vi "Coral Controller.vi"(3 "error in":errorcluster) -> ()   [LabVIEW 2023]
doc: "This VI executes continuously carrying out the current operation and responding to updates or new operations. It will often contain the timing or control code that is difficult to place directly in TeleOp. This VI generally opens all sensors and motors and isolates the rest of the robot code from knowing how the operations are carried out."
uses:
  <vilib>/Rock Robotics/WPI/Framework/Completion Status.ctl
  Coral Setpoints.ctl
  Coral Operations.ctl
  Support Code/Teleop Util/Coral States.ctl
  Support Code/Teleop Util/Scoring Levels.ctl
  <vilib>/Rock Robotics/WPI/ThirdParty/REV Robotics/REVLib/Typedef/Spark MAX Idle Mode.ctl
  <vilib>/Rock Robotics/WPI/ThirdParty/REV Robotics/REVLib/Typedef/SPARK Closed Loop Slot.ctl
  <vilib>/Rock Robotics/SystemInterfaces/DIO/FPGA_DIOChannel.ctl
  <vilib>/Rock Robotics/WPI/ThirdParty/REV Robotics/REVLib/Typedef/Spark MAX Control Type.ctl
  da023379-89e9-4f2e-8a2f-b1c80103741f.vi
  <vilib>/Rock Robotics/WPI/ThirdParty/REV Robotics/REVLib/SubVI/Public/SPARK Open Brushless.vi
  <vilib>/Rock Robotics/WPI/ThirdParty/REV Robotics/REVLib/SubVI/Public/SPARK Configure Basic Idle Mode.vi
  <vilib>/Rock Robotics/WPI/ThirdParty/REV Robotics/REVLib/SubVI/Public/SPARK Configure Basic Inverted.vi
  <vilib>/Rock Robotics/WPI/ThirdParty/REV Robotics/REVLib/SubVI/Public/SPARK Configure Encoder Conversion Factors.vi
  <vilib>/Rock Robotics/WPI/ThirdParty/REV Robotics/REVLib/SubVI/Public/SPARK Configure Limit Switch Reverse.vi
  <vilib>/Rock Robotics/WPI/ThirdParty/REV Robotics/REVLib/SubVI/Public/SPARK Configure Soft Limit Forward.vi
  <vilib>/Rock Robotics/WPI/ThirdParty/REV Robotics/REVLib/SubVI/Public/SPARK Configure Soft Limit Reverse.vi
  <vilib>/Rock Robotics/WPI/ThirdParty/REV Robotics/REVLib/SubVI/Public/SPARK Configure Power Smart Current Limit.vi
  <vilib>/Rock Robotics/WPI/ThirdParty/REV Robotics/REVLib/SubVI/Public/SPARK Configure Closed Loop Miscellaneous.vi
  <vilib>/Rock Robotics/Network Tables/NT Write String.vi
  Framework/Robot Global Data.vi
  <vilib>/Rock Robotics/Network Tables/NT Read Number.vi
  <vilib>/Rock Robotics/WPI/ThirdParty/REV Robotics/REVLib/SubVI/Public/SPARK Get Encoder Status Position.vi
  <vilib>/Rock Robotics/WPI/ThirdParty/REV Robotics/REVLib/SubVI/Public/SPARK Get Device Status Output Current.vi
  <vilib>/Rock Robotics/WPI/ThirdParty/REV Robotics/REVLib/SubVI/Public/SPARK Get Encoder Status Velocity.vi
  <vilib>/Rock Robotics/Network Tables/NT Write Number.vi
  <vilib>/Rock Robotics/WPI/ThirdParty/REV Robotics/REVLib/Typedef/Spark MAX Limit Switch Polarity.ctl
  <vilib>/Rock Robotics/WPI/ThirdParty/REV Robotics/REVLib/SubVI/Public/SPARK Configure Limit Switch Forward.vi
  <vilib>/Rock Robotics/Network Tables/NT Write Boolean.vi
  <vilib>/Rock Robotics/WPI/ThirdParty/REV Robotics/REVLib/SubVI/Public/SPARK Configure Follower Mode From Ref.vi
panel:
  out "Detect DIO0?":bool=TRUE
  in  "sensor speed launcher 2":dbl=850.0
  out "Coral Seen":dbl(graph)
  out "Detect DIO2?":bool=TRUE
  out "Detect DIO1?":bool=TRUE
  in  "Arbitrary Feed Forward (0)":dbl=0.7
  out "End Time":dbl=0.4
  out "Current":dbl(graph)=11.245421245421245
  in  "Trapezoid Fly off?":bool
  out "Grounded Trapezoid":cluster{"Sensor Velocity":dbl, "Numeric":dbl}[](graph)=[{"Sensor Velocity"=-0.075857974588871, "Numeric"=0.0}, {"Sensor Velocity"=-0.0156947523355484, "Numeric"=300.0}, {"Sensor Velocity"=-1.0724748373031616, "Numeric"=600.0}, {"Sensor Velocity"=6.980241298675537, "Numeric"=900.0}, {"Sensor Velocity"=67.09114837646484, "Numeric"=1200.0}, {"Sensor Velocity"=197.5812530517578, "Numeric"=1500.0}, {"Sensor Velocity"=419.5848388671875, "Numeric"=1800.0}, {"Sensor Velocity"=710.8807983398438, "Numeric"=2100.0}, {"Sensor Velocity"=1095.191650390625, "Numeric"=2400.0}, {"Sensor Velocity"=1497.837890625, "Numeric"=2700.0}, {"Sensor Velocity"=1889.49267578125, "Numeric"=3000.0}, {"Sensor Velocity"=2250.2314453125, "Numeric"=2947.8500604629517}, {"Sensor Velocity"=2563.325927734375, "Numeric"=2647.8500604629517}, {"Sensor Velocity"=2824.191162109375, "Numeric"=2347.8500604629517}, {"Sensor Velocity"=3000.52685546875, "Numeric"=2047.8500604629512}, {"Sensor Velocity"=2896.772705078125, "Numeric"=1747.850060462952}, {"Sensor Velocity"=2896.772705078125, "Numeric"=1447.8500604629517}, {"Sensor Velocity"=2564.4833984375, "Numeric"=1147.8500604629512}, {"Sensor Velocity"=2022.881103515625, "Numeric"=847.8500604629517}, {"Sensor Velocity"=1387.4384765625, "Numeric"=547.8500604629517}, {"Sensor Velocity"=826.7198486328125, "Numeric"=247.8500604629512}, {"Sensor Velocity"=386.8534240722656, "Numeric"=0.0}, {"Sensor Velocity"=110.9880599975586, "Numeric"=0.0}]
  out "Sensor Experiment":bool
  out "Post-Trapezoid Sensor Position":dbl=-9.590681076049805
  out "Scoring Sequence Trapezoid":cluster{"Sensor Velocity":dbl, "Numeric":dbl}[](graph)=[{"Sensor Velocity"=0.0, "Numeric"=-0.0}, {"Sensor Velocity"=-7.134573459625244, "Numeric"=-300.0}, {"Sensor Velocity"=-7.134573459625244, "Numeric"=-600.0}, {"Sensor Velocity"=-41.63425827026367, "Numeric"=-900.0}, {"Sensor Velocity"=-125.5266342163086, "Numeric"=-1200.0}, {"Sensor Velocity"=-259.8109436035156, "Numeric"=-1500.0}, {"Sensor Velocity"=-446.01348876953125, "Numeric"=-1800.0}, {"Sensor Velocity"=-687.0809936523438, "Numeric"=-2100.0}, {"Sensor Velocity"=-1302.1033935546875, "Numeric"=-2400.0}, {"Sensor Velocity"=-1302.1033935546875, "Numeric"=-2700.0}, {"Sensor Velocity"=-1660.494384765625, "Numeric"=-3000.0}, {"Sensor Velocity"=-1997.8662109375, "Numeric"=-2704.006862640381}, {"Sensor Velocity"=-2354.501953125, "Numeric"=-2404.006862640381}, {"Sensor Velocity"=-2687.039794921875, "Numeric"=-2104.006862640381}, {"Sensor Velocity"=-2901.859130859375, "Numeric"=-1804.0068626403804}, {"Sensor Velocity"=-2966.857666015625, "Numeric"=-1504.006862640381}, {"Sensor Velocity"=-2838.606689453125, "Numeric"=-1204.0068626403809}, {"Sensor Velocity"=-1969.9622802734375, "Numeric"=-904.0068626403804}, {"Sensor Velocity"=-1969.9622802734375, "Numeric"=-604.0068626403809}, {"Sensor Velocity"=-1384.843505859375, "Numeric"=-304.00686264038086}, {"Sensor Velocity"=-874.3311767578125, "Numeric"=0.0}, {"Sensor Velocity"=-466.64947509765625, "Numeric"=0.0}]
  in  "Acceleration Max":dbl=15000.0
  in  "Velocity Max":dbl=5000.0
  out "Coral Seen":dbl
  out "Velocity Chart for Tuning":dbl(graph)=920.4789428710938
  in  "Launcher PID":T1={"P Gain"=0.0, "I Gain"=1e-06, "D Gain"=0.0, "F Gain"=0.0001, "I Zone"=0.0, "Min Output"=-0.5, "Max Output"=0.5}
  in  "Max I Accum":dbl=100.0
  in  "L4 PID Constant":T1={"P Gain"=0.0, "I Gain"=0.0, "D Gain"=0.0, "F Gain"=0.0, "I Zone"=0.0, "Min Output"=-0.8, "Max Output"=0.8}
  in  "coral threshold":dbl=10.0
  in  "Distance Decrease Grounded":dbl
  out "Command Timing":u32(graph)=7
  in  "Distance Decrease":dbl
  out "Intake Trapezoid Chart":cluster{"Sensor Velocity":dbl, "Numeric":dbl}[](graph)
  out "Position Chart (All Time)":cluster{"Sensor Position":dbl}(graph)={"Sensor Position"=-0.0436662957072258}
  out "Post Position Correction":dbl=-9.5556640625
  out "detect?":bool
  in  "sensor speed launcher":dbl=1250.0
  in  "launcher speed":dbl=1250.0
  in  "FF multiplier":dbl=0.39
  out "Pivot Chart":T2(graph)={"Sensor Velocity"=-4.928565979003906, "Arbitrary Feedforward"=-6.429}
  in  "Velocity PID Test":T1={"P Gain"=0.0002, "I Gain"=0.0, "D Gain"=0.0, "F Gain"=0.000165, "I Zone"=0.0, "Min Output"=-1.0, "Max Output"=1.0}
  in  "Positional PID Test":T1={"P Gain"=0.07, "I Gain"=0.0, "D Gain"=0.0, "F Gain"=0.0, "I Zone"=0.0, "Min Output"=-0.6, "Max Output"=0.6}
  in  "Intake Pivot Test":T1={"P Gain"=0.09, "I Gain"=0.0, "D Gain"=0.0, "F Gain"=-0.0, "I Zone"=0.0, "Min Output"=-0.8, "Max Output"=0.8}
  in  "detected speed (0)":dbl
  in  "FeedForward Constants":cluster{"kA":dbl, "kS":dbl, "kG":dbl, "kV":dbl}={"kA"=0.0, "kS"=0.0, "kG"=-0.57, "kV"=0.0}
  in  "intake setpoint":dbl=-0.95
  in  "Interactive Values":T3
  out "Current\nCmd":string="Started at  07:33:49.500\n: Immediate,  CS Grounded, SS Default"
  in  "Buttons":cluster{"Execute Cmd":bool, "Abort Cmd":bool}
  out "Command Timing":cluster{"Start Time (ms)":u32, "Iterations":i32}={"Start Time (ms)"=1054953, "Iterations"=0}
  out "Status":T7=enum."Aborted"
  # "old value 1250"
  # "irrelevant for now"
  # "sarah wuz here\nreasonable terms\nriyasonable terms"
  # "luke was here(maybe idk anymore)"
  # "intake speed: must be negative"
  # "launchee speed when intaking"
  # "Interactive Command: You may fill in the settings for a command\nand schedule it with the Execute button. You can observe and abort\nany command while fine tuning the code for the controller."
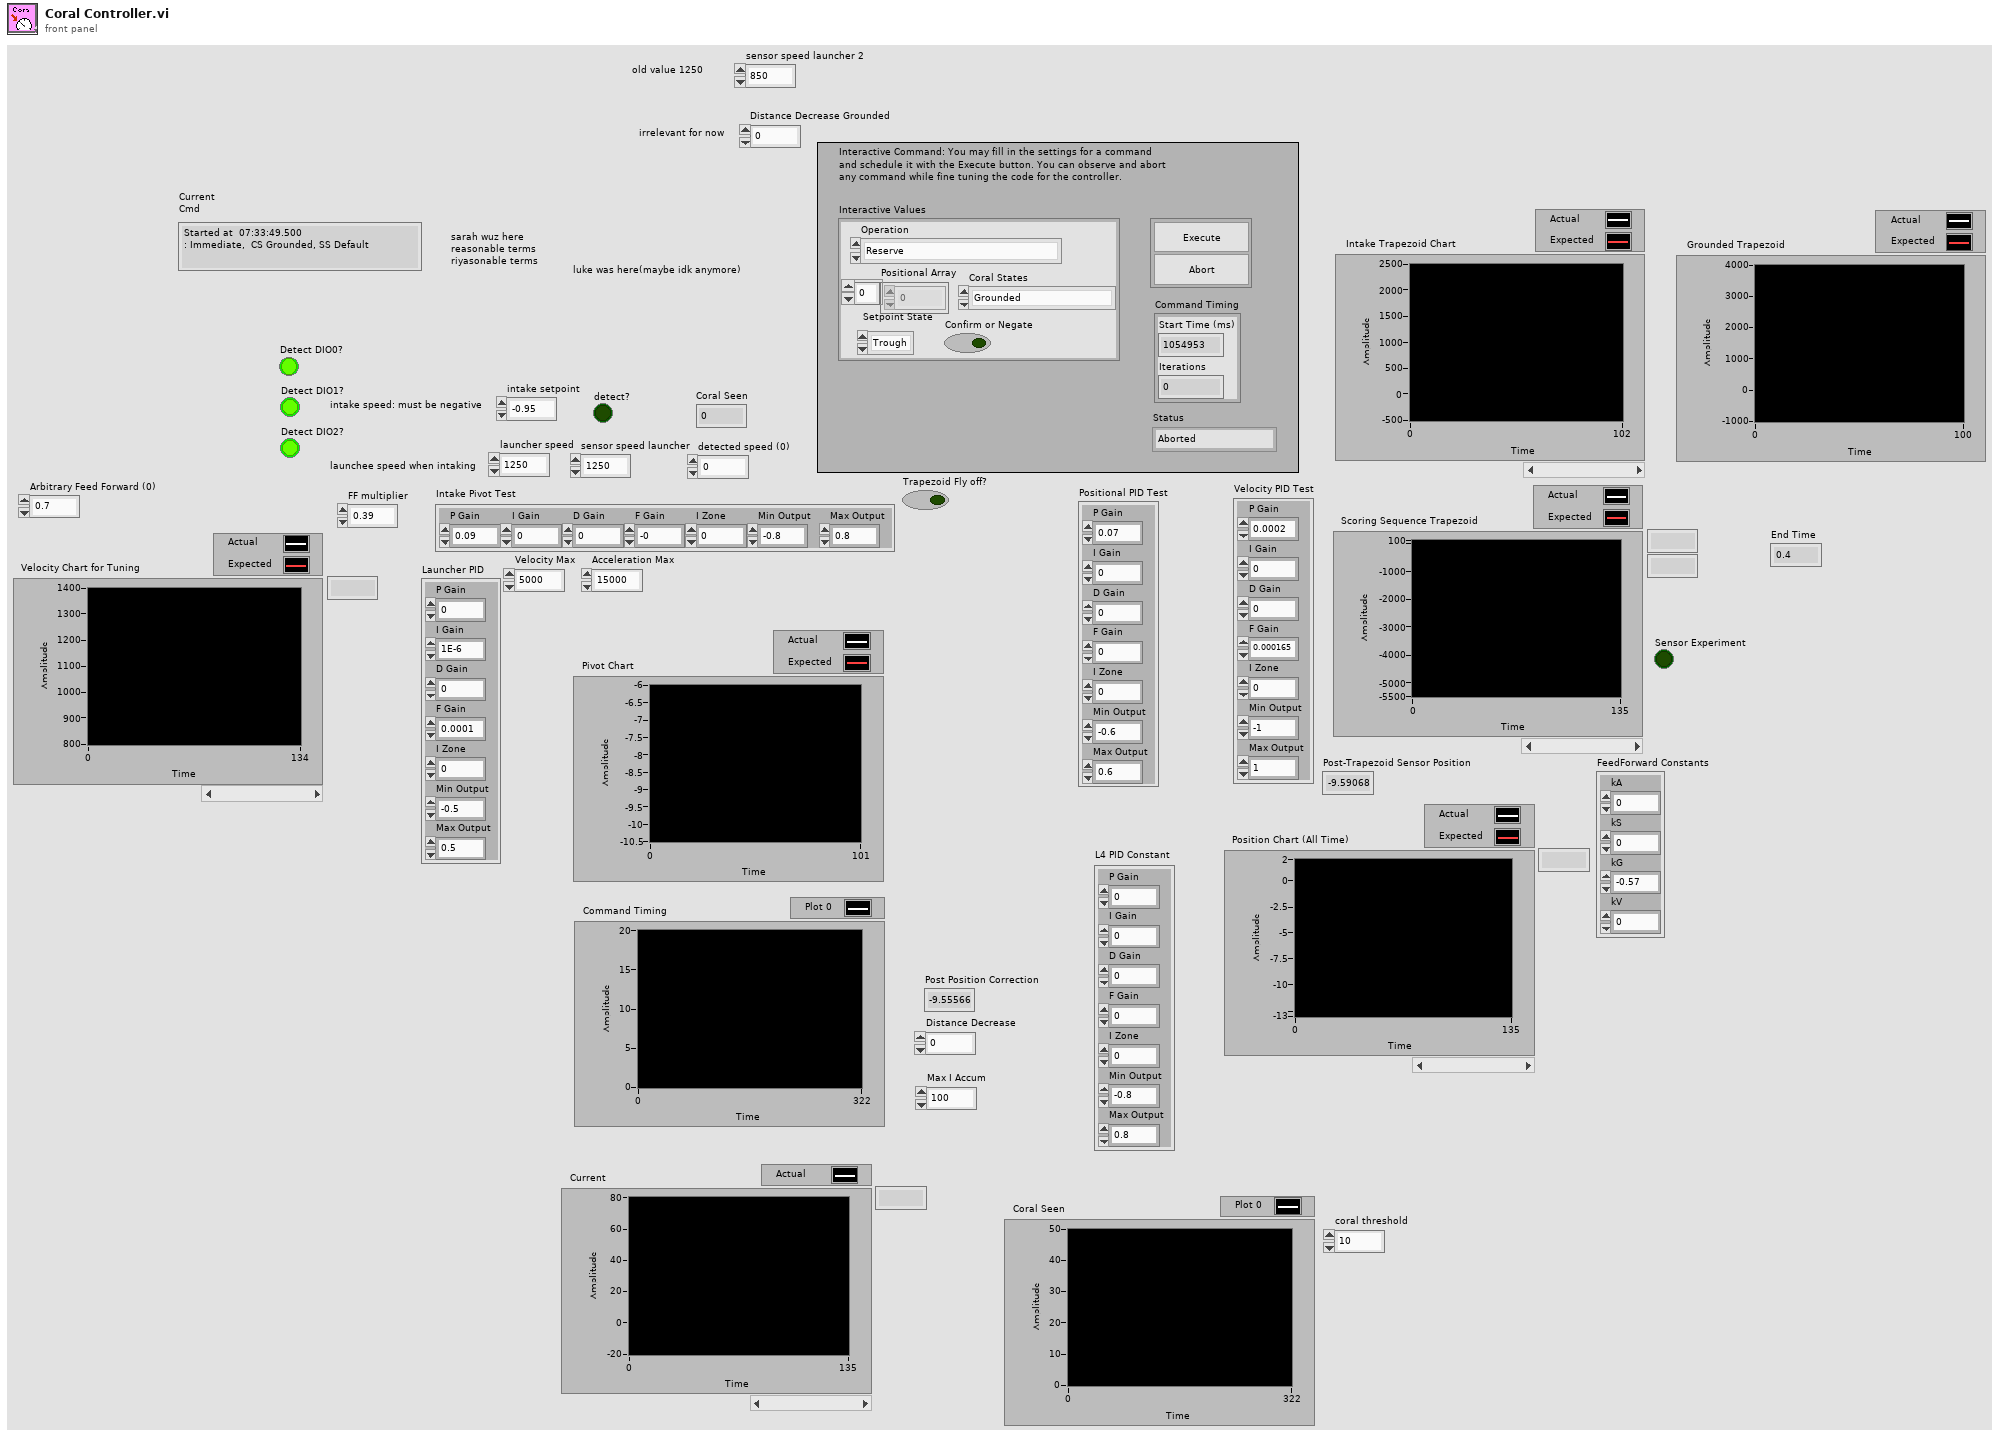
[diagram p1: front panel]
types:
  T1 = cluster{"P Gain":dbl, "I Gain":dbl, "D Gain":dbl, "F Gain":dbl, "I Zone":dbl, "Min Output":dbl, "Max Output":dbl}
  T2 = cluster{"Sensor Velocity":dbl, "Arbitrary Feedforward":dbl}
  T3 = typedef "Coral Setpoints.ctl" = cluster{"Operation":T4, "Coral States":T5, "Confirm or Negate":bool, "Positional Array":dbl[], "Setpoint State":T6}
  T4 = typedef "Coral Operations.ctl" = enum16{"Reserve", "Read Current", "Immediate", "Calibrate"}
  T5 = typedef "Coral States.ctl" = enum16{"Grounded", "Coral Intake", "Scoring Sequence", "Hold Position", "Score", "Manual Override", "Climb Safety Mode"}
  T6 = typedef "Scoring Levels.ctl" = enum16{"Trough", "L2", "L3", "L4", "Default"}
  T7 = typedef "Completion Status.ctl" = enum16{"Successful", "Aborted", "Incomplete"}
  T8 = typedef "FPGA_DIOChannel.ctl" = enum8{"DIO 0", "DIO 1", "DIO 2", "DIO 3", "DIO 4", "DIO 5", "DIO 6", "DIO 7", "DIO 8", "DIO 9", "DIO MXP 0", "DIO MXP 1", "DIO MXP 2", "DIO MXP 3", "DIO MXP 4", "DIO MXP 5", "DIO MXP 6", "DIO MXP 7", "DIO MXP 8", "DIO MXP 9", "DIO MXP 10", "DIO MXP 11", "DIO MXP 12", "DIO MXP 13", "DIO MXP 14", "DIO MXP 15", "SPI Port CS1", "SPI Port CS2", "SPI Port CS3", "SPI Port MISO", "SPI Port MOSI", "Invalid"}
  T9 = typedef "Spark MAX Idle Mode.ctl" = enum16{"Coast", "Brake"}
  T10 = typedef "SPARK Closed Loop Slot.ctl" = u16
  T11 = typedef "WPI_MotorControlDeviceRef.ctl" = cluster{"DeviceStatus":errorcluster, "Type":T12, "PWM":cluster{"PWM Channel":T13, "DeadBand":T14}, "CAN":cluster{"Device Number":u8, "SetOutput VI Ref":variant, "GetOutput VI Ref":variant, "Enable VI Ref":variant, "Disable VI Ref":variant, "Data":variant}, "Invert":bool, "DIO PWM":cluster{"PWM \"Enable\" Channel":T13, "DIOChannel":T8, "PWM Rate":dbl}}
  T12 = typedef "WPI_MotorControlType.ctl" = enum16{"PWM", "CAN", "DIO PWM"}
  T13 = typedef "FPGA_DIOPWMChannel.ctl" = enum8{"PWM 0", "PWM 1", "PWM 2", "PWM 3", "PWM 4", "PWM 5", "PWM 6", "PWM 7", "PWM 8", "PWM 9", "PWM MXP 0", "PWM MXP 1", "PWM MXP 2", "PWM MXP 3", "PWM MXP 4", "PWM MXP 5", "PWM MXP 6", "PWM MXP 7", "PWM MXP 8", "PWM MXP 9", "Invalid"}
  T14 = typedef "WPI_PWMDeadband.ctl" = cluster{"Name":string, "maxPositivePwm":i32, "minPositivePwm":i32, "centerPwm":i32, "maxNegativePwm":i32, "minNegativePwm":i32, "angularRange":u16}
  T15 = typedef "Command Status Info.ctl" = cluster{"Name":string, "Status":T7, "notifier out":T16}
  T16 = typedef "Completion Notifier.ctl" = refnum<notifier>
  T17 = typedef "WPI_DigitalInputDevRef.ctl" = cluster{"DevStatus":errorcluster, "DIO Channel":T8}
  T18 = cluster{"Current Command":T3, "Command Timing":cluster{"Start Time (ms)":u32, "Iterations":i32}, "Command Arguments":cluster{"Command Info":T15, "Description":string, "Default Command":T3, "queue out":refnum<queue>, "Subsystem Name":string}}
  T19 = typedef "Spark MAX Control Type.ctl" = enum16{"Percent VBus", "Voltage", "Velocity", "Position", "Smart Motion", "Current", "Smart Velocity", "MAXMotion Position", "MAXMotion Velocity"}
  T20 = typedef "Spark MAX Limit Switch Polarity.ctl" = enum16{"Normally Open", "Normally Closed"}
  T21 = cluster{"Setpoint Configs":cluster{"Scoring Setpoint":T6, "Position Setpoint":dbl, "Trapezoid":dbl[], "Score Power":dbl}[]}
  T22 = cluster{"Scoring Setpoint":T6, "Position Setpoint":dbl, "Trapezoid":dbl[], "Score Power":dbl}[]
  T23 = cluster{"Scoring Setpoint":T6, "Position Setpoint":dbl, "Trapezoid":dbl[], "Score Power":dbl}
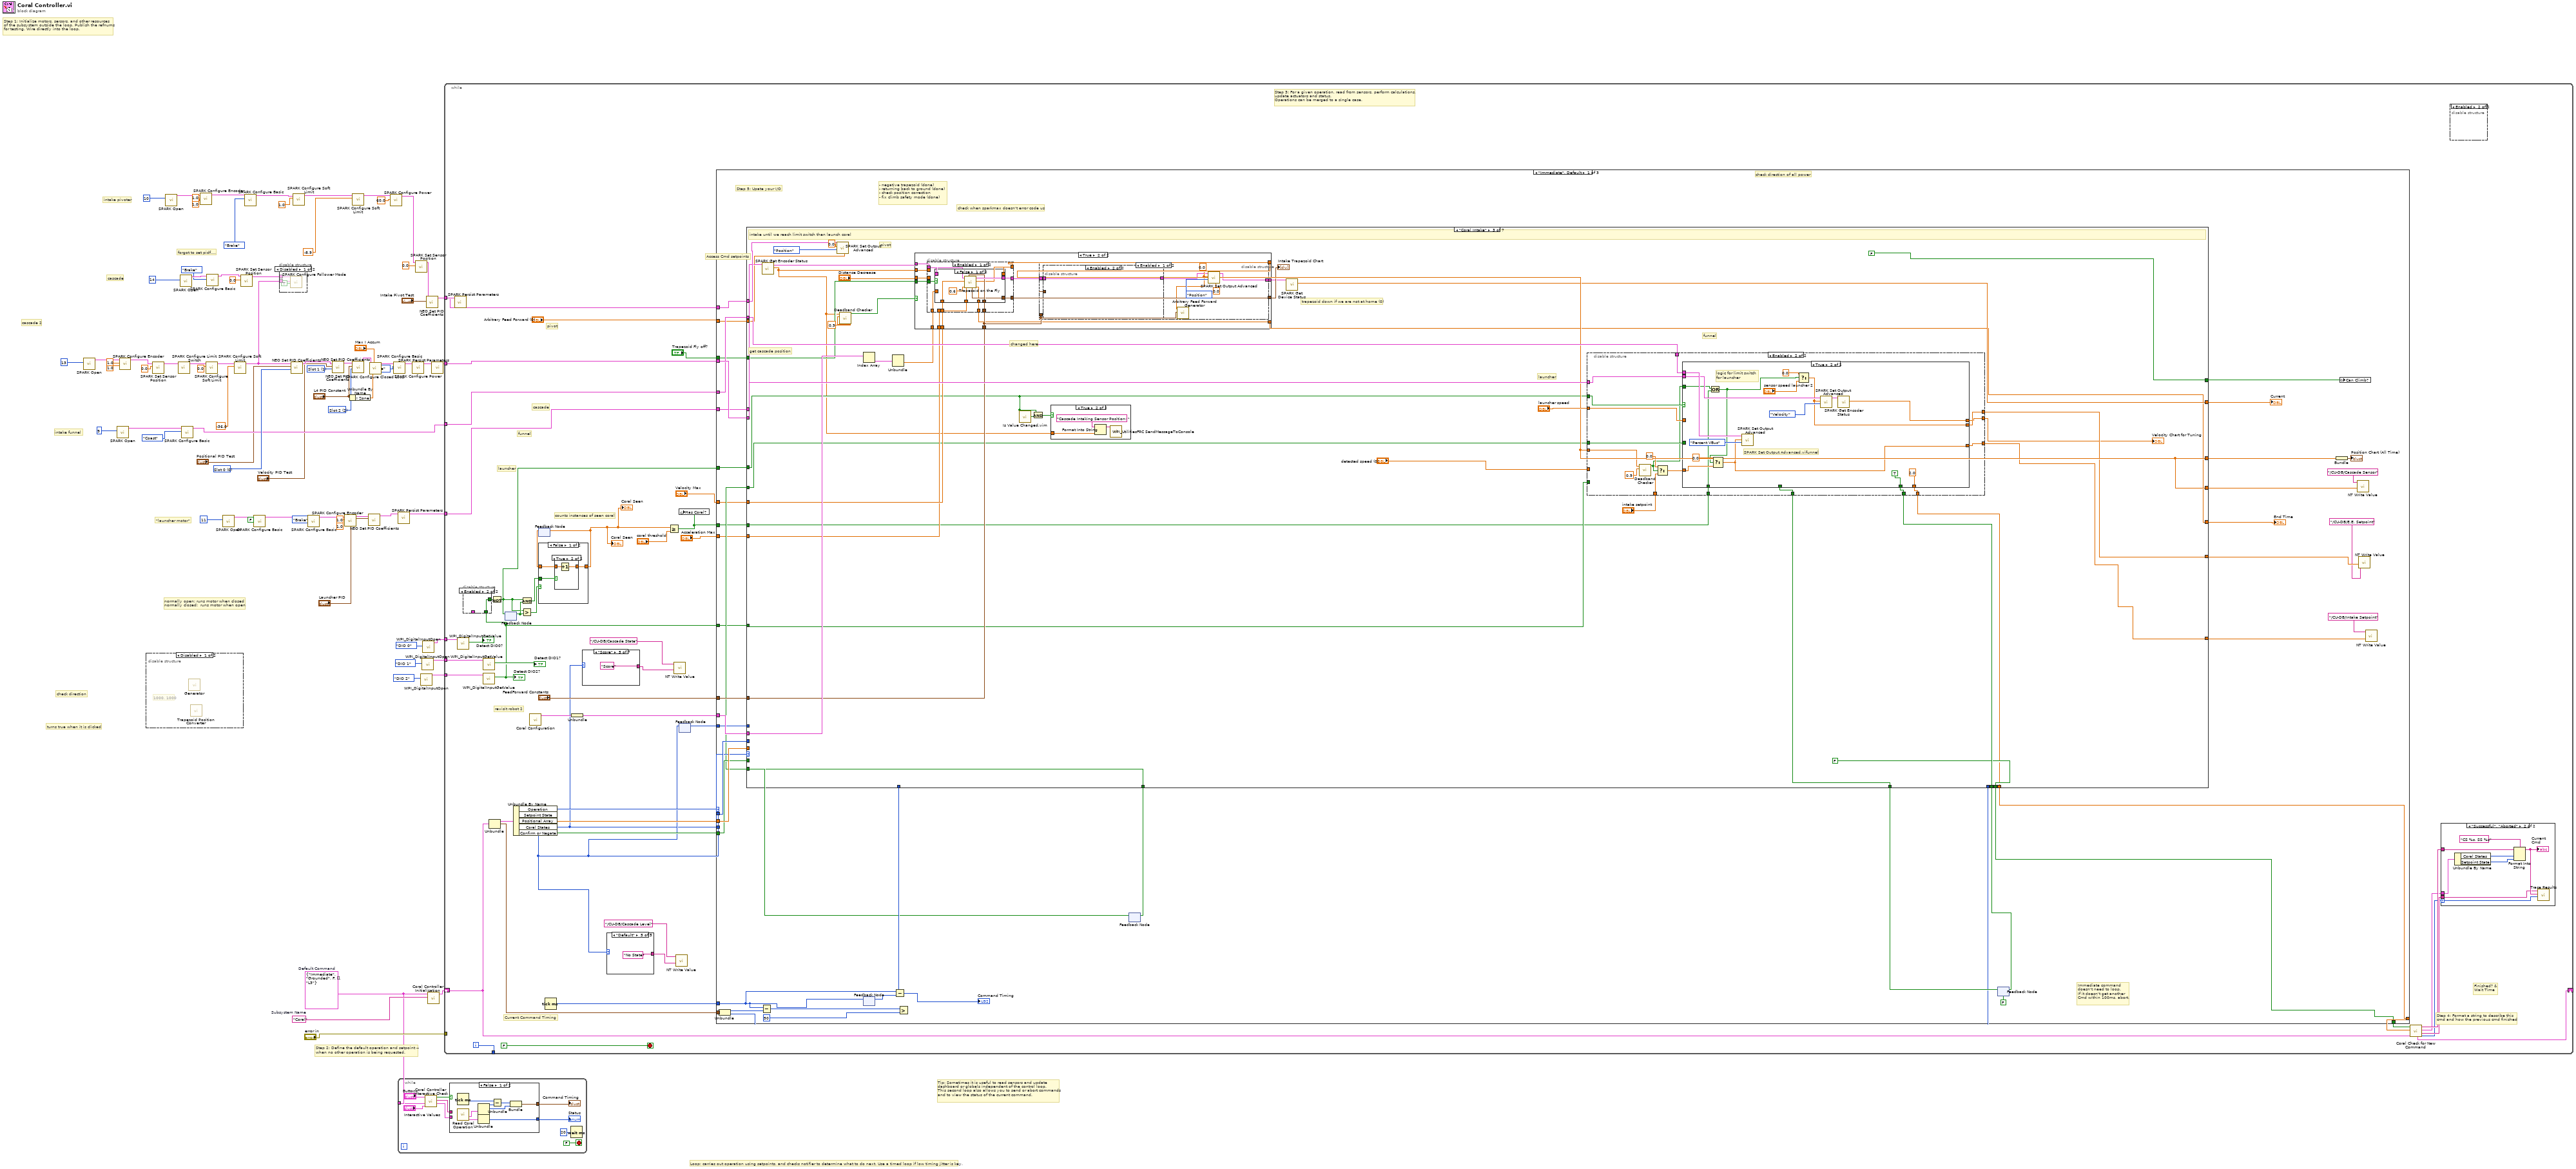
[diagram p0: block diagram]
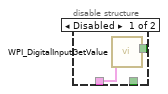
[diagram p2: hidden frame]
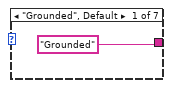
[diagram p3: hidden frame]
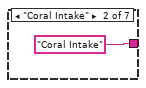
[diagram p4: hidden frame]
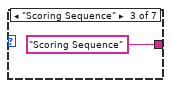
[diagram p5: hidden frame]
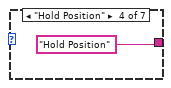
[diagram p6: hidden frame]
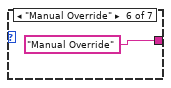
[diagram p7: hidden frame]
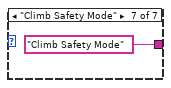
[diagram p8: hidden frame]
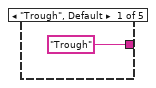
[diagram p9: hidden frame]
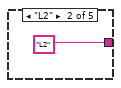
[diagram p10: hidden frame]
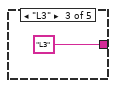
[diagram p11: hidden frame]
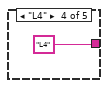
[diagram p12: hidden frame]
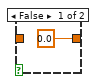
[diagram p13: hidden frame]
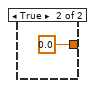
[diagram p14: hidden frame]
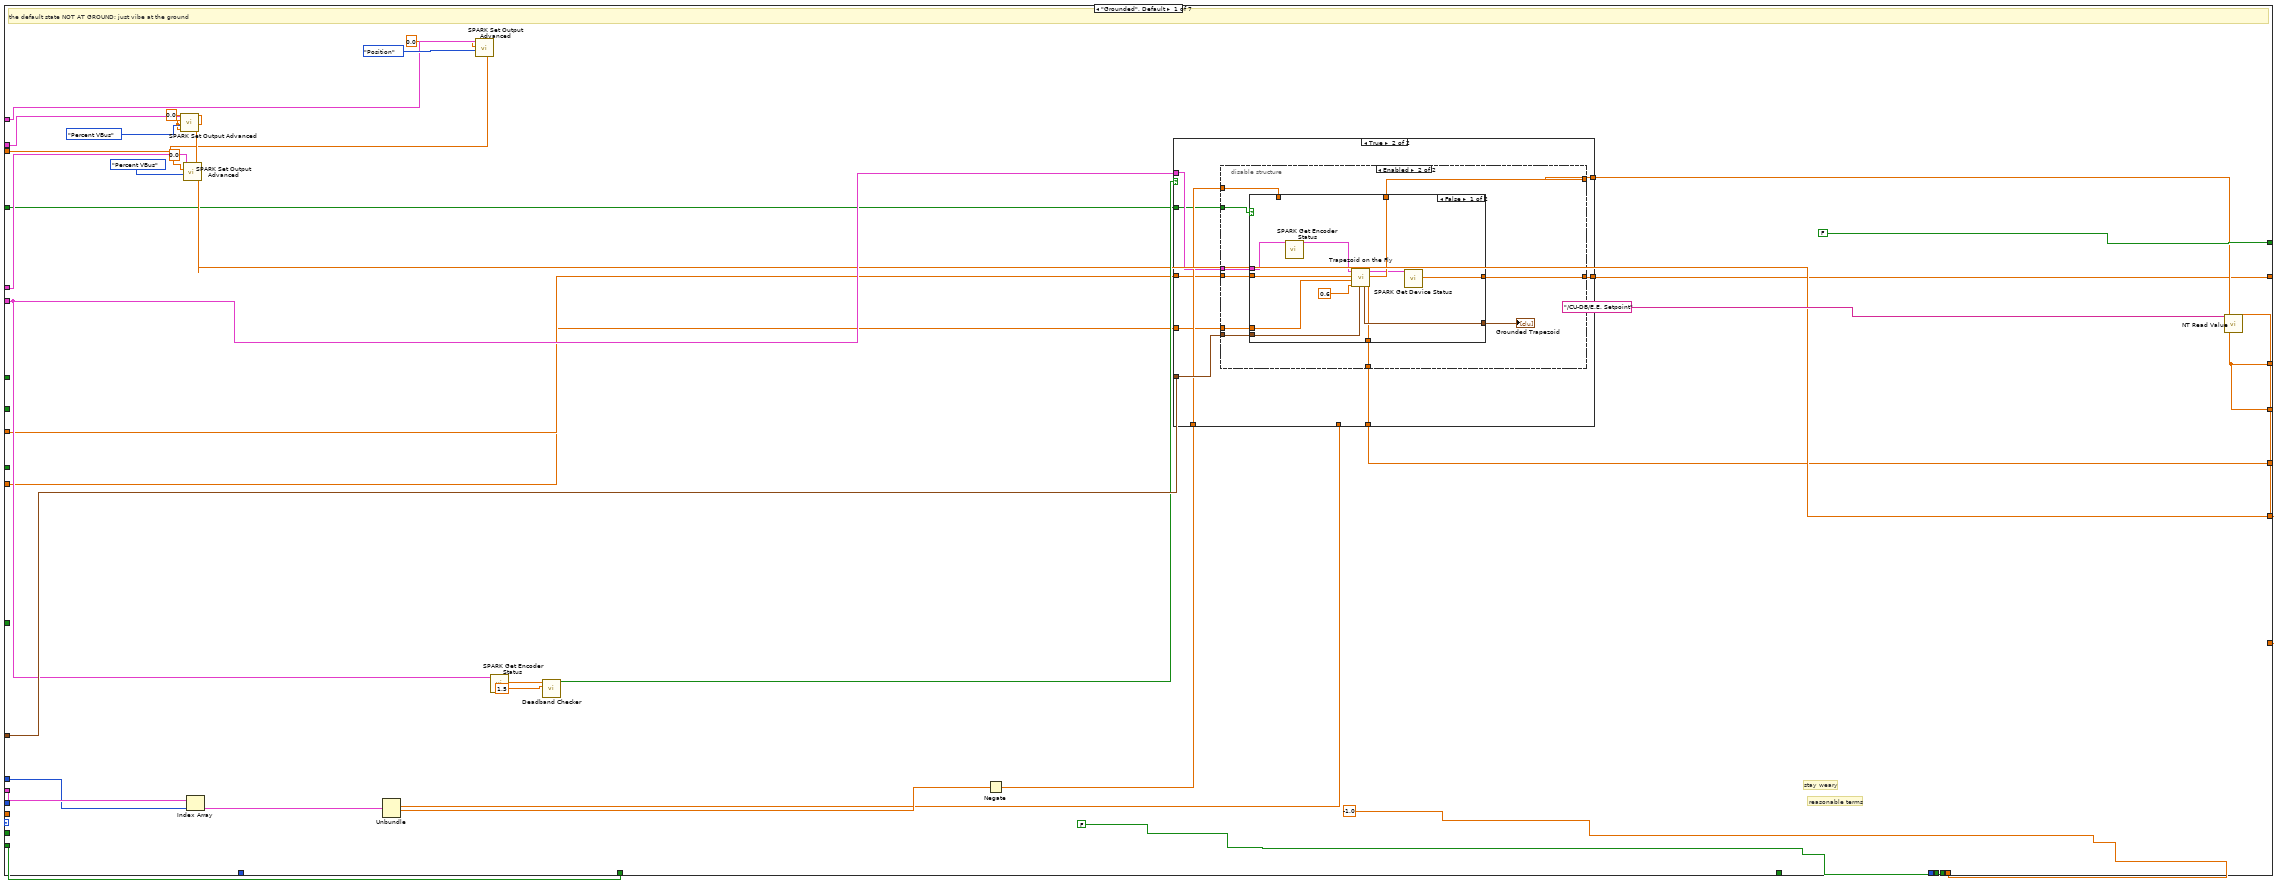
[diagram p15: hidden frame]
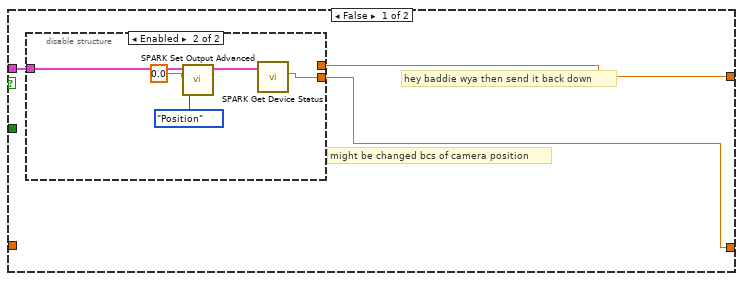
[diagram p16: hidden frame]
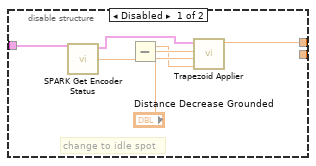
[diagram p17: hidden frame]
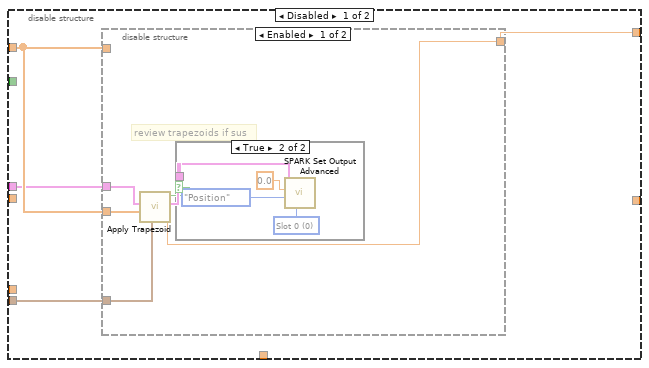
[diagram p18: hidden frame]
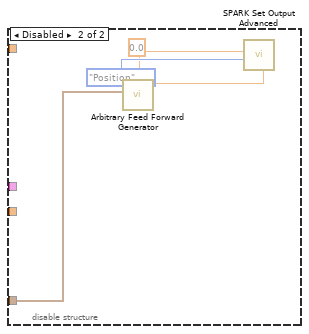
[diagram p20: hidden frame]
diagram:
  (unwired) 1.0 ("Velocity Conversion Factor")
  w18 = T10 2 items=["Slot 0", "Slot 1", "Slot 2", "Slot 3"] ("Loop Slot")
  w58 = T10 1 items=["Slot 0", "Slot 1", "Slot 2", "Slot 3"] ("Loop Slot")
  w60 = T10 0 items=["Slot 0", "Slot 1", "Slot 2", "Slot 3"] ("Loop Slot")
  w74 = T3 {"Operation"=enum."Immediate", "Coral States"=enum."Grounded", "Confirm or Negate"=FALSE, "Positional Array"=[], "Setpoint State"=enum."L3"}  # Default Command
  w75 = "Coral"  # Subsystem Name
  # "intake pivoter"
  # "intake funnel"
  # "cascade 2"
  # "cascade"
  # "turns true when it is clicked"
  # "normally open: runs motor when closed\nnormally closed:  runs motor when open"
  # "check direction"
  # "\"launcher motor\""
  # "forgot to set pidf...."
  # "Tip: Sometimes it is useful to read sensors and update\ndashboard or globals independent of the control loop.\nThis second loop also allows you to send or abort commands\nand to view the status of the current command."
  # "Step 2: Define the default operation and setpoint --\nwhen no other operation is being requested."
  # "Step 1: Initialize motors, sersors, and other resources\nof the subsystem outside the loop. Publish the refnums\nfor testing. Wire directly into the loop."
  # "Loop: carries out operation using setpoints, and checks notifier to determine what to do next. Use a timed loop if low timing jitter is key."
  n1 = call-poly <vilib>:"SPARK Open.vi"("Device Number"=u8 13) -> ("MotorControlDeviceRef"=w68:T11)  [unwired: 9 in, 1 out]
  n2 = call-poly <vilib>:"SPARK Open.vi"("Device Number"=u8 9) -> ("MotorControlDeviceRef"=w50:T11)  [unwired: 9 in, 1 out]
  n3 = call-poly <vilib>:"SPARK Configure Encoder.vi"("Velocity Conversion Factor"=1.0, "Position Conversion Factor"=1.0, "MotorControlDeviceRef in"=w68) -> ("MotorControlDeviceRef out"=w32:T11)  [unwired: 7 in, 1 out]
  n4 = disable-structure shown="Disabled" {
    frame Disabled {
      # "1000, 1000"
      n5 = call "Generator.vi"() -> ("Velocity Max"=w78:dbl, "Acceleration Max"=w79:dbl)  [unwired: 8 in, 2 out]
      n6 = call "Trapezoid Position Converter.vi"() -> ()  [unwired: 11 in, 1 out]
    }
    frame Enabled {
    }
  }
  n7 = call <vilib>:"SPARK Set Sensor Position.vi"("Position"=0.0, "MotorControlDeviceRef"=w32) -> ("MotorControlDeviceRef"=w67:T11)  [unwired: 8 in, 1 out]
  n8 = call-poly <vilib>:"SPARK Open.vi"("Device Number"=u8 10) -> ("MotorControlDeviceRef"=w29:T11)  [unwired: 9 in, 1 out]
  n9 = call-poly <vilib>:"SPARK Configure Limit Switch.vi"("MotorControlDeviceRef in"=w67) -> ("MotorControlDeviceRef out"=w65:T11)  [unwired: 9 in, 1 out]
  n10 = call-poly <vilib>:"SPARK Open.vi"("Device Number"=u8 14) -> ("MotorControlDeviceRef"=w5:T11)  [unwired: 9 in, 1 out]
  n11 = call-poly <vilib>:"SPARK Configure Basic.vi"("Idle Mode"=Spark_MAX_Idle_Mode."Coast", "MotorControlDeviceRef in"=w50) -> ("MotorControlDeviceRef out"=w49:T11)  [unwired: 8 in, 1 out]
  n12 = call-poly <vilib>:"SPARK Configure Encoder.vi"("Velocity Conversion Factor"=1.0, "Position Conversion Factor"=1.0, "MotorControlDeviceRef in"=w29) -> ("MotorControlDeviceRef out"=w28:T11)  [unwired: 7 in, 1 out]
  n13 = call-poly <vilib>:"SPARK Configure Soft Limit.vi"("Soft Limit"=0.0, "MotorControlDeviceRef in"=w65) -> ("MotorControlDeviceRef out"=w71:T11)  [unwired: 8 in, 1 out]
  n14 = call-poly <vilib>:"SPARK Configure Basic.vi"("Idle Mode"=Spark_MAX_Idle_Mode."Brake", "MotorControlDeviceRef in"=w5) -> ("MotorControlDeviceRef out"=w3:T11)  [unwired: 8 in, 1 out]
  n15 = call-poly <vilib>:"SPARK Open.vi"("Device Number"=u8 11) -> ("MotorControlDeviceRef"=w57:T11)  [unwired: 9 in, 1 out]
  n16 = call-poly <vilib>:"SPARK Configure Soft Limit.vi"("Soft Limit"=-36.0, "MotorControlDeviceRef in"=w71) -> ("MotorControlDeviceRef out"=w73:T11)  [unwired: 8 in, 1 out]
  n17 = call <vilib>:"SPARK Set Sensor Position.vi"("Position"=0.0, "MotorControlDeviceRef"=w3) -> ("MotorControlDeviceRef"=w55:T11)  [unwired: 8 in, 1 out]
  n18 = call-poly <vilib>:"SPARK Configure Basic.vi"("Idle Mode"=Spark_MAX_Idle_Mode."Brake", "MotorControlDeviceRef in"=w28) -> ("MotorControlDeviceRef out"=w52:T11)  [unwired: 8 in, 1 out]
  n19 = call-poly <vilib>:"SPARK Configure Basic.vi"("Inverted (F)"=FALSE, "MotorControlDeviceRef in"=w57) -> ("MotorControlDeviceRef out"=w43:T11)  [unwired: 8 in, 1 out]
  n20 = disable-structure shown="Disabled" {
    disable-tunnel: w55 -> [w82 _]
    disable-tunnel: w73 -> [w81 _]
    frame Disabled {
      n21 = call-poly <vilib>:"SPARK Configure Follower Mode.vi"("Invert From Leader"=TRUE, "Leader MotorControlDeviceRef"=w81, "MotorControlDeviceRef in"=w82) -> ()  [unwired: 7 in, 2 out]
    }
    frame Enabled {
    }
  }
  n22 = call "NEO Set PID Coefficients.vi"("Closed Loop Slot"=w60, "PID Constants"="Positional PID Test", "MotorControlDeviceRef in"=w73) -> ("MotorControlDeviceRef out"=w59:T11)  [unwired: 5 in, 1 out]
  n23 = call-poly <vilib>:"SPARK Configure Soft Limit.vi"("Soft Limit"=1.0, "MotorControlDeviceRef in"=w52) -> ("MotorControlDeviceRef out"=w54:T11)  [unwired: 8 in, 1 out]
  n24 = call-poly <vilib>:"SPARK Configure Basic.vi"("Idle Mode"=Spark_MAX_Idle_Mode."Brake", "MotorControlDeviceRef in"=w43) -> ("MotorControlDeviceRef out"=w9:T11)  [unwired: 8 in, 1 out]
  n25 = call "NEO Set PID Coefficients.vi"("Closed Loop Slot"=w58, "PID Constants"="Velocity PID Test", "MotorControlDeviceRef in"=w59) -> ("MotorControlDeviceRef out"=w19:T11)  [unwired: 5 in, 1 out]
  n26 = call-poly <vilib>:"SPARK Configure Encoder.vi"("Position Conversion Factor"=1.0, "MotorControlDeviceRef in"=w9) -> ("MotorControlDeviceRef out"=w8:T11)  [unwired: 8 in, 1 out]
  n27 = Unbundle By Name("L4 PID Constant") -> ("I Zone"=w13:dbl)
  n28 = call-poly <vilib>:"SPARK Configure Soft Limit.vi"("Soft Limit"=-8.9, "MotorControlDeviceRef in"=w54) -> ("MotorControlDeviceRef out"=w51:T11)  [unwired: 8 in, 1 out]
  n29 = call "NEO Set PID Coefficients.vi"("Closed Loop Slot"=w18, "PID Constants"="L4 PID Constant", "MotorControlDeviceRef in"=w19) -> ("MotorControlDeviceRef out"=w17:T11)  [unwired: 5 in, 1 out]
  n30 = call "NEO Set PID Coefficients.vi"("PID Constants"="Launcher PID", "MotorControlDeviceRef in"=w8) -> ("MotorControlDeviceRef out"=w12:T11)  [unwired: 6 in, 1 out]
  n31 = call-poly <vilib>:"SPARK Configure Closed Loop.vi"("Max I Accum"="Max I Accum", "I Zone"=w13, "MotorControlDeviceRef in"=w17) -> ("MotorControlDeviceRef out"=w16:T11)  [unwired: 7 in, 1 out]
  n32 = call-poly <vilib>:"SPARK Configure Power.vi"("Primay Current Limit (80A)"=60.0, "MotorControlDeviceRef in"=w51) -> ("MotorControlDeviceRef out"=w35:T11)  [unwired: 8 in, 1 out]
  n33 = call-poly <vilib>:"SPARK Configure Basic.vi"("Idle Mode"=Spark_MAX_Idle_Mode."Brake", "MotorControlDeviceRef in"=w16) -> ("MotorControlDeviceRef out"=w63:T11)  [unwired: 8 in, 1 out]
  n34 = while {
    tunnel: w74 -> [w89]
    stop <- FALSE stop-if-true
    n35 = call "Coral Controller Interactive Check.vi"("Interactive Command in"="Interactive Values", "Default Command"=w89, "Buttons"="Buttons") -> ("Interactive Command out"=w86:T3, "Trace String"=w87:string, "Schedule"=w88:bool)  [unwired: 6 in]
    n36 = case shown="False" w88 {
      tunnel: [w100 w105] -> w85
      tunnel: w86 -> [_ w103]
      tunnel: [w96 w101] -> w84
      tunnel: w87 -> [_ w104]
      frame False {
        n37 = Tick Count (ms)() -> (millisecond timer value=w95:u32)
        n38 = call "Read Coral Operation.vi"() -> ("Command Info"=w93:T15, "SubSystem Data"=w94:T3)  [unwired: 9 in, 1 out]
        n39 = Unbundle(w94) -> ("Operation"=w99:T4, "Coral States"=w97:T5)  [unwired: 3 out]
        n40 = Unbundle(w93) -> ("Status"=w100:T7)  [unwired: 2 out]
        n41 = Subtract(x=w95, y=w99) -> (x-y=w98:u32)
        n42 = Bundle(w98, "Coral States"=w97) -> (w96:cluster{u32, "Coral States":T5})  [unwired: 1 in]
      }
      frame True {
        n43 = call "Coral Command Helper.vi"("Description"=w104, "SubSystem Data"=w103) -> ("Command Info Out"=w102:T15, "Command Timing"=w101:cluster{"Start Time (ms)":u32, "Iterations":i32})  [unwired: 7 in, 1 out]
        n44 = Unbundle(w102) -> ("Status"=w105:T7)  [unwired: 2 out]
      }
    }
    "Status" <- w85
    "Command Timing" <- w84
    n45 = Wait (ms)(milliseconds to wait=u32 20) -> ()  [unwired: 1 out]
  }
  n46 = call <vilib>:"SPARK Persist Parameters.vi"("MotorControlDeviceRef"=w12) -> ("MotorControlDeviceRef"=w20:T11)  [unwired: 9 in, 1 out]
  n47 = call-poly <vilib>:"SPARK Configure Power.vi"("MotorControlDeviceRef in"=w63) -> ("MotorControlDeviceRef out"=w22:T11)  [unwired: 9 in, 1 out]
  n48 = call <vilib>:"SPARK Set Sensor Position.vi"("Position"=0.0, "MotorControlDeviceRef"=w35) -> ("MotorControlDeviceRef"=w25:T11)  [unwired: 8 in, 1 out]
  n49 = call <vilib>:"WPI_DigitalInputOpen.vi"("DIO Channel"=FPGA_DIOChannel."DIO 2") -> ("DigitalInputDevRef"=w1:T17)  [unwired: 9 in, 1 out]
  n50 = call <vilib>:"WPI_DigitalInputOpen.vi"("DIO Channel"=FPGA_DIOChannel."DIO 1") -> ("DigitalInputDevRef"=w6:T17)  [unwired: 9 in, 1 out]
  n51 = call <vilib>:"WPI_DigitalInputOpen.vi"("DIO Channel"=FPGA_DIOChannel."DIO 0") -> ("DigitalInputDevRef"=w39:T17)  [unwired: 9 in, 1 out]
  n52 = call "NEO Set PID Coefficients.vi"("PID Constants"="Intake Pivot Test", "MotorControlDeviceRef in"=w25) -> ("MotorControlDeviceRef out"=w34:T11)  [unwired: 6 in, 1 out]
  n53 = call "Coral Controller Initialization.vi"("Subsystem Name"=w75, "Default Command"=w74) -> ("Current Command"=w76:T18)  [unwired: 9 in]
  n54 = call <vilib>:"SPARK Persist Parameters.vi"("MotorControlDeviceRef"=w22) -> ("MotorControlDeviceRef"=w21:T11)  [unwired: 9 in, 1 out]
  n55 = call <vilib>:"SPARK Persist Parameters.vi"("MotorControlDeviceRef"=w34) -> ("MotorControlDeviceRef"=w23:T11)  [unwired: 9 in, 1 out]
  n56 = while {
    shift-right: [w147] -> _
    shift-left: w76 -> [w140]
    tunnel: [w153] -> _
    tunnel: "error in" -> [_]
    tunnel: w49 -> [w138]
    tunnel: w20 -> [w139]
    tunnel: w21 -> [w132]
    tunnel: w39 -> [w107]
    tunnel: w23 -> [w133]
    tunnel: w6 -> [w115]
    tunnel: w1 -> [w112]
    i -> [w153]
    stop <- FALSE stop-if-true
    # "counts instances of seen coral"
    # "pivot"
    # "funnel"
    # "cascade"
    # "launcher"
    # "revisit robot 2"
    # "Step 5: Upate your I/O"
    # "Step 4: Format a string to describe this\ncmd and how the previous cmd finished"
    # "Current Command Timing"
    # "Access Cmd setpoints"
    # "Finished? &\nWait Time"
    # "Step 3: For a given operation, read from sensors, perform calculations,\nupdate actuators and status.\nOperations can be merged to a single case."
    n57 = call <vilib>:"WPI_DigitalInputGetValue.vi"("DigitalInputDevRef"=w107) -> ("Value"=→"Detect DIO0?":bool)  [unwired: 8 in, 2 out]
    n58 = call <vilib>:"WPI_DigitalInputGetValue.vi"("DigitalInputDevRef"=w112) -> ("Value"=w109:bool)  [unwired: 8 in, 2 out]
    "Detect DIO2?" <- w109
    n59 = disable-structure shown="Enabled" {
      disable-tunnel: [w156 w157] -> w131
      disable-tunnel: _ -> [w155 _]
      disable-tunnel: w109 -> [_ w157]
      frame Disabled {
        n60 = call <vilib>:"WPI_DigitalInputGetValue.vi"("DigitalInputDevRef"=w155) -> ("Value"=w156:bool)  [unwired: 8 in, 2 out]
      }
      frame Enabled {
      }
    }
    n61 = call <vilib>:"WPI_DigitalInputGetValue.vi"("DigitalInputDevRef"=w115) -> ("Value"=→"Detect DIO1?":bool)  [unwired: 8 in, 2 out]
    n62 = Unbundle(w140) -> ("Current Command"=w152:T3, "Command Timing"=w149:cluster{"Start Time (ms)":u32, "Iterations":i32})  [unwired: 1 out]
    n63 = Not(x=w131) -> (.not. x?=w118:bool)
    n64 = feedback-in #1(w118) -> ()
    n65 = feedback #1() -> (w130:bool)  [unwired: 1 in]
    n66 = Unbundle By Name(w152) -> ("Operation"=w151:T4, "Setpoint State"=w122:T6, "Positional Array"=w148:dbl[], "Coral States"=w121:T5, "Confirm or Negate"=w137:bool)
    n67 = Greater?(x=w118, y=w130) -> (0:w129:bool)
    n68 = And(x=w118, y=w130) -> (x .and. y?=w127:bool)
    n69 = call "Coral Configuration.vi"() -> ("Coral Config"=w136:T21)  [unwired: 10 in, 1 out]
    n70 = feedback #2() -> (w128:dbl)  [unwired: 1 in]
    n71 = case shown="False" w129 {
      tunnel: [w170 0.0] -> w111
      tunnel: w128 -> [w171 _]
      tunnel: w127 -> [w172 _]
      frame False {
        n72 = case shown="True" w172 {
          tunnel: w171 -> [_ w175]
          tunnel: [0.0 w174] -> w170
          frame False {
          }
          frame True {
            n73 = Increment(x=w175) -> (x+1=w174:dbl)
          }
        }
      }
      frame True {
      }
    }
    "Coral Seen" <- w111
    "Coral Seen" <- w111
    n74 = feedback-in #2(w111) -> ()
    n75 = Tick Count (ms)() -> (millisecond timer value=w150:u32)
    n76 = Unbundle(w136) -> ("Setpoint Configs"=w134:T22)
    n77 = case shown="\"Score\"" w121 {
      tunnel: ["Grounded" "Coral Intake" "Scoring Sequence" "Hold Position" "Score" "Manual Override" "Climb Safety Mode"] -> w120
      frame "Grounded", Default {
      }
      frame "Coral Intake" {
      }
      frame "Scoring Sequence" {
      }
      frame "Hold Position" {
      }
      frame "Score" {
      }
      frame "Manual Override" {
      }
      frame "Climb Safety Mode" {
      }
    }
    n78 = case shown="\"Default\"" w122 {
      tunnel: ["Trough" "L2" "L3" "L4" "No State"] -> w125
      frame "Trough", Default {
      }
      frame "L2" {
      }
      frame "L3" {
      }
      frame "L4" {
      }
      frame "Default" {
      }
    }
    n79 = Greater Or Equal?(x=w111, y="coral threshold") -> (x >= y?=w108:bool)
    n80 = call-poly <vilib>:"NT Write Value.vi"("value"=w120, "name"="/CU-DB/Cascade State") -> ()  [unwired: 9 in, 1 out]
    n81 = call-poly <vilib>:"NT Write Value.vi"("value"=w125, "name"="/CU-DB/Cascade Level") -> ()  [unwired: 9 in, 1 out]
    n82 = global write "Robot Global Data.vi" "Has Coral?"(w108) -> ()
    n83 = feedback-in #3(w122) -> ()
    n84 = feedback #3() -> (w123:T6)  [unwired: 1 in]
    n85 = case shown="\"Immediate\", Default" w151 {
      tunnel: [w204 -1.0 ("Infinite") w860] -> w145
      tunnel: [w203 FALSE ("ignore previous (F)") FALSE ("ignore previous (F)")] -> w146
      tunnel: w149 -> [w217 _ _]
      tunnel: w122 -> [w210 _ _]
      tunnel: w150 -> [w196 _ _]
      tunnel: w148 -> [w214 _ _]
      tunnel: w121 -> [w209 _ _]
      tunnel: w132 -> [w216 w844 w855]
      tunnel: w139 -> [w215 w835 w854]
      tunnel: w138 -> [w212 w838 w849]
      tunnel: w137 -> [w213 _ _]
      tunnel: w133 -> [w211 w839 w845]
      tunnel: "FeedForward Constants" -> [w208 _ _]
      tunnel: w134 -> [w202 _ _]
      tunnel: w123 -> [w194 _ _]
      tunnel: w118 -> [w187 _ _]
      tunnel: "Velocity Max" -> [w184 _ _]
      tunnel: "Acceleration Max" -> [w183 _ _]
      tunnel: "Trapezoid Fly off?" -> [w182 _ _]
      tunnel: "Arbitrary Feed Forward (0)" -> [w179 _ _]
      tunnel: w109 -> [w178 _ _]
      tunnel: w108 -> [w177 _ _]
      frame "Immediate", Default {
        # "- negative trapezoid (done)\n- returning back to ground (done)\n- check position correction\n- fix climb safety mode (done)"
        # "check when sparkmax doesn't error code us"
        # "check direction of all power"
        # "Immediate command\ndoesn't need to loop.\nIf it doesn't get another\nCmd within 100ms, abort."
        n86 = Unbundle(w217) -> ("Start Time (ms)"=w220:u32, "Iterations"=w195:i32)
        n87 = Subtract(x=w196, y=w220) -> (x-y=w219:u32)
        n88 = feedback-in #4(w196) -> ()
        n89 = feedback #4() -> (w199:u32)  [unwired: 1 in]
        n90 = Subtract(x=w196, y=w199) -> (x-y=→"Command Timing":u32)
        n91 = Greater?(x=w219, y=u8 50 ("Left Motor")) -> ()  [unwired: 1 out]
        n92 = feedback #5() -> (w185:bool)  [unwired: 1 in]
        n93 = feedback #6(FALSE) -> (w205:bool)
        n94 = case shown="\"Coral Intake\"" w209 {
          tunnel: w216 -> [w238 w365 w418 w679 w769 w800 w831]
          tunnel: w215 -> [w251 w351 w421 w681 w766 _ _]
          tunnel: w214 -> [_ _ _ _ _ _ _]
          tunnel: w213 -> [_ _ _ _ _ w799 _]
          tunnel: w210 -> [_ _ _ w668 w771 _ w820]
          tunnel: w202 -> [w243 _ w404 w667 w772 _ w821]
          tunnel: w212 -> [w253 w349 w425 w684 _ _ _]
          tunnel: w211 -> [w248 w348 w424 w675 _ _ w830]
          tunnel: w208 -> [w246 w336 w400 w678 w776 w796 w828]
          tunnel: [FALSE ("Boolean") FALSE ("Boolean") FALSE ("Boolean") FALSE ("Boolean") FALSE ("Boolean") FALSE ("Boolean") FALSE ("Boolean")] -> w203
          tunnel: [FALSE w354 FALSE FALSE FALSE FALSE FALSE] -> w207
          tunnel: [w245 w353 w420 w674 FALSE w794 w824] -> w206
          tunnel: w205 -> [w245 w353 w419 w674 _ w794 w824]
          tunnel: [-1.0 ("Infinite") 20.0 ("Infinite") w410 20.0 ("Infinite") 20.0 ("Infinite") 20.0 ("Infinite") 20.0 ("Infinite")] -> w204
          tunnel: [w232 0.0 w407 w664 w763 w787 w815] -> w201
          tunnel: w196 -> [_ _ _ _ _ _ _]
          tunnel: w195 -> [_ _ _ _ _ _ _]
          tunnel: w194 -> [w233 _ _ w658 _ _ _]
          tunnel: [w232 nan w407 w664 w763 w787 w815] -> w192
          tunnel: [w230 w342 w406 w662 w762 w785 w813] -> w191
          tunnel: [w229 w344 w405 0.0 w760 w783 w811] -> w188
          tunnel: w187 -> [_ _ w386 w642 _ _ w810]
          tunnel: [w228 w343 w399 w641 w759 TRUE w807] -> w186
          tunnel: w185 -> [_ _ w389 _ _ _ w808]
          tunnel: w185 -> [w228 w343 w399 _ w759 _ w807]
          tunnel: w184 -> [w227 w338 w398 w649 _ _ _]
          tunnel: w183 -> [w226 w339 w397 w650 _ _ _]
          tunnel: w182 -> [w224 _ w396 w647 _ _ _]
          tunnel: [w223 w340 w393 w645 w757 w780 w805] -> w181
          tunnel: [w222 _ w392 w644 _ _ _] -> w180
          tunnel: w179 -> [w221 _ w391 w643 _ _ w804]
          tunnel: w178 -> [_ _ w390 _ _ _ _]
          tunnel: w177 -> [_ _ w388 _ _ _ _]
          frame "Grounded", Default {
            w229 = 0.0 ("Setpoint")
            # "reasonable terms"
            # "stay weary"
            # "the default state NOT AT GROUND; just vibe at the ground"
            n95 = call <vilib>:"SPARK Set Output Advanced.vi"("Control Mode"=Spark_MAX_Control_Type."Percent VBus", "Setpoint"=w229, "MotorControlDevRef"=w253) -> ()  [unwired: 7 in, 2 out]
            n96 = call <vilib>:"SPARK Set Output Advanced.vi"("Control Mode"=Spark_MAX_Control_Type."Percent VBus", "Setpoint"=0.0, "MotorControlDevRef"=w251) -> ()  [unwired: 7 in, 2 out]
            n97 = Index Array(array=w243, index=w233) -> (element=w242:T23)
            n98 = Unbundle(w242) -> ("Position Setpoint"=w225:dbl, "Trapezoid"=w234:dbl[])  [unwired: 2 out]
            n99 = call <vilib>:"SPARK Set Output Advanced.vi"("Arbitrary Feed Forward (0)"=w221, "Control Mode"=Spark_MAX_Control_Type."Position", "Setpoint"=0.0 ("t"), "MotorControlDevRef"=w248) -> ()  [unwired: 6 in, 2 out]
            n100 = call-poly <vilib>:"SPARK Get Encoder Status.vi"("MotorControlDevRef in"=w238) -> ("Sensor Position"=w236:dbl)  [unwired: 7 in, 3 out]
            n101 = call "Deadband Checker.vi"("Limit"=1.5, "Value"=w236) -> ("Outside Deadband?"=w237:bool)  [unwired: 9 in]
            n102 = Negate(x=w234) -> (-x=w247:dbl[])
            n103 = case shown="True" w237 {
              tunnel: w238 -> [w256 w276]
              tunnel: w247 -> [_ w277]
              tunnel: w246 -> [_ w278]
              tunnel: [w257 w275] -> w232
              tunnel: w227 -> [_ w274]
              tunnel: w226 -> [_ w273]
              tunnel: w225 -> [_ _]
              tunnel: w224 -> [_ w272]
              tunnel: [w255 w271] -> w223
              tunnel: [_ w270] -> w222
              frame False {
                # "might be changed bcs of camera position"
                # "hey baddie wya then send it back down"
                n104 = disable-structure shown="Enabled" {
                  disable-tunnel: [w264 _] -> w257
                  disable-tunnel: w256 -> [w263 w269]
                  disable-tunnel: [_ w265] -> w255
                  frame Disabled {
                    # "change to idle spot"
                    n105 = call-poly <vilib>:"SPARK Get Encoder Status.vi"("MotorControlDevRef in"=w263) -> ("Sensor Position"=w262:dbl, "MotorControlDevRef out"=w260:T11)  [unwired: 7 in, 2 out]
                    n106 = Subtract(x=w258, y=w262) -> (x-y=w261:dbl)
                    n107 = call "Trapezoid Applier.vi"("Distance Decrease"="Distance Decrease Grounded", "Distance to Setpoint"=w261, "MotorControlDevRef in"=w260) -> ("Sensor Position out"=w264:dbl, "Intended Position"=w258:dbl)  [unwired: 6 in, 1 out]
                  }
                  frame Enabled {
                    n108 = call <vilib>:"SPARK Set Output Advanced.vi"("Control Mode"=Spark_MAX_Control_Type."Position", "Setpoint"=0.0, "MotorControlDevRef"=w269) -> ("MotorControlDevRef"=w266:T11)  [unwired: 7 in, 1 out]
                    n109 = call-poly <vilib>:"SPARK Get Device Status.vi"("MotorControlDevRef in"=w266) -> ("Current"=w265:dbl)  [unwired: 7 in, 3 out]
                  }
                }
              }
              frame True {
                n110 = disable-structure shown="Enabled" {
                  disable-tunnel: w278 -> [w282 w306]
                  disable-tunnel: w277 -> [w281 w303]
                  disable-tunnel: w276 -> [w280 w304]
                  disable-tunnel: [w279 w305] -> w275
                  disable-tunnel: w274 -> [_ w308]
                  disable-tunnel: w273 -> [_ w307]
                  disable-tunnel: w272 -> [_ w302]
                  disable-tunnel: [_ w301] -> w271
                  disable-tunnel: [_ w299] -> w270
                  frame Disabled {
                    n111 = disable-structure shown="Enabled" {
                      disable-tunnel: w281 -> [_ _]
                      disable-tunnel: w282 -> [w289 w295]
                      disable-tunnel: w281 -> [w287 _]
                      disable-tunnel: w280 -> [w286 _]
                      disable-tunnel: [w285 _] -> w279
                      frame Enabled {
                        # "review trapezoids if sus"
                        n112 = call "Apply Trapezoid.vi"("FeedForward Constants"=w289, "Velocity values"=w287, "MotorControlDeviceRef in"=w286) -> ("Sensor Position"=w285:dbl, "MotorControlDevRef out"=w284:T11, "Boolean"=w283:bool, "charted V"=w288:cluster{"Sensor Velocity":dbl, "Numeric":dbl}[])  [unwired: 5 in]
                        n113 = case shown="True" w283 {
                          tunnel: w284 -> [_ w293]
                          frame False {
                          }
                          frame True {
                            w290 = T10 0 items=["Slot 0", "Slot 1", "Slot 2", "Slot 3"] ("Closed Loop Slot")
                            n114 = call <vilib>:"SPARK Set Output Advanced.vi"("Closed Loop Slot"=w290, "Control Mode"=Spark_MAX_Control_Type."Position", "Setpoint"=0.0, "MotorControlDevRef"=w293) -> ()  [unwired: 6 in, 2 out]
                          }
                        }
                      }
                      frame Disabled {
                        w294 = 0.0 ("Setpoint")
                        n115 = call "Arbitrary Feed Forward Generator.vi"("Feed Forward Constants"=w295, "Setpoint"=w294) -> ("Arbitrary Feedforward"=w296:dbl)  [unwired: 9 in]
                        n116 = call <vilib>:"SPARK Set Output Advanced.vi"("Arbitrary Feed Forward (0)"=w296, "Control Mode"=Spark_MAX_Control_Type."Position", "Setpoint"=w294) -> ("MotorControlDevRef"=w297:T11)  [unwired: 6 in, 2 out]
                      }
                    }
                  }
                  frame Enabled {
                    n117 = case shown="False" w302 {
                      tunnel: w308 -> [w319 _]
                      tunnel: w307 -> [w318 _]
                      tunnel: w306 -> [w317 w322]
                      tunnel: [w316 w325] -> w305
                      tunnel: w304 -> [w314 w324]
                      tunnel: w303 -> [_ w323]
                      tunnel: [w312 w321] -> w301
                      tunnel: [w311 w320] -> w300
                      tunnel: [w310 _] -> w299
                      frame False {
                        n118 = call-poly <vilib>:"SPARK Get Encoder Status.vi"("MotorControlDevRef in"=w314) -> ("MotorControlDevRef out"=w315:T11)  [unwired: 7 in, 3 out]
                        n119 = call "Trapezoid on the Fly.vi"("FeedForward Constants"=w317, "Setpoint"=0.6, "Acceleration Max"=w318, "Velocity Max"=w319, "MotorControlDevRef in"=w315) -> ("End Time"=w310:dbl, "Sensor Position"=w316:dbl, "MotorControlDevRef out"=w313:T11, "charted V"=w311:cluster{"Sensor Velocity":dbl, "Numeric":dbl}[])  [unwired: 1 out]
                        n120 = call-poly <vilib>:"SPARK Get Device Status.vi"("MotorControlDevRef in"=w313) -> ("Current"=w312:dbl)  [unwired: 7 in, 3 out]
                      }
                      frame True {
                        # "review trapezoids if sus"
                        n121 = call "Apply Trapezoid.vi"("FeedForward Constants"=w322, "Velocity values"=w323, "MotorControlDeviceRef in"=w324) -> ("Sensor Position"=w325:dbl, "MotorControlDevRef out"=w327:T11, "Boolean"=w326:bool, "charted V"=w320:cluster{"Sensor Velocity":dbl, "Numeric":dbl}[])  [unwired: 5 in]
                        n122 = case shown="False" w326 {
                          tunnel: w327 -> [w329 w335]
                          tunnel: [w328 w330] -> w321
                          frame False {
                            n123 = call-poly <vilib>:"SPARK Get Device Status.vi"("MotorControlDevRef in"=w329) -> ("Current"=w328:dbl)  [unwired: 7 in, 3 out]
                          }
                          frame True {
                            w332 = T10 0 items=["Slot 0", "Slot 1", "Slot 2", "Slot 3"] ("Closed Loop Slot")
                            n124 = call <vilib>:"SPARK Set Output Advanced.vi"("Closed Loop Slot"=w332, "Control Mode"=Spark_MAX_Control_Type."Position", "Setpoint"=0.0, "MotorControlDevRef"=w335) -> ("MotorControlDevRef"=w331:T11)  [unwired: 6 in, 1 out]
                            n125 = call-poly <vilib>:"SPARK Get Device Status.vi"("MotorControlDevRef in"=w331) -> ("Current"=w330:dbl)  [unwired: 7 in, 3 out]
                          }
                        }
                      }
                    }
                    "Grounded Trapezoid" <- w300
                  }
                }
              }
            }
            n126 = call-poly <vilib>:"NT Read Value.vi"("name"="/CU-DB/E.E. Setpoint") -> ("value"=w230:dbl)  [unwired: 8 in, 2 out]
          }
          frame "Climb Safety Mode" {
            w362 = -6.429 ("Setpoint")
            w342 = 0.0 ("Setpoint")
            w344 = 0.0 ("Setpoint")
            # "pivot intake out of the way and do not move any motors on intake so we do not crash into climb"
            n127 = disable-structure shown="Enabled" {
              disable-tunnel: w365 -> [w367 w378]
              disable-tunnel: w339 -> [_ w373]
              disable-tunnel: w338 -> [_ w372]
              disable-tunnel: 0.0 ("Setpoint") -> [_ w371]
              disable-tunnel: w336 -> [_ w370]
              frame Enabled {
                n128 = call <vilib>:"SPARK Set Output Advanced.vi"("Control Mode"=Spark_MAX_Control_Type."Percent VBus", "Setpoint"=0.0, "MotorControlDevRef"=w367) -> ()  [unwired: 7 in, 2 out]
              }
              frame Disabled {
                n129 = call-poly <vilib>:"SPARK Get Encoder Status.vi"("MotorControlDevRef in"=w378) -> ("Sensor Position"=w374:dbl, "MotorControlDevRef out"=w377:T11)  [unwired: 7 in, 2 out]
                n130 = call "Deadband Checker.vi"("Limit"=1.5, "Value"=w374) -> ("Outside Deadband?"=w375:bool)  [unwired: 9 in]
                n131 = case shown="True" w375 {
                  tunnel: w377 -> [_ w383]
                  tunnel: w373 -> [_ w382]
                  tunnel: w372 -> [_ w381]
                  tunnel: w371 -> [_ w380]
                  tunnel: w370 -> [_ w379]
                  frame False {
                  }
                  frame True {
                    n132 = call "Trapezoid on the Fly.vi"("FeedForward Constants"=w379, "Setpoint"=w380, "Acceleration Max"=w382, "Velocity Max"=w381, "MotorControlDevRef in"=w383) -> ()  [unwired: 5 out]
                  }
                }
              }
            }
            n133 = call <vilib>:"SPARK Set Output Advanced.vi"("Control Mode"=Spark_MAX_Control_Type."Percent VBus", "Setpoint"=w342, "MotorControlDevRef"=w351) -> ("MotorControlDevRef"=w341:T11)  [unwired: 7 in, 1 out]
            n134 = call-poly <vilib>:"SPARK Get Encoder Status.vi"("MotorControlDevRef in"=w348) -> ("Sensor Position"=w356:dbl, "MotorControlDevRef out"=w347:T11)  [unwired: 7 in, 2 out]
            n135 = call-poly <vilib>:"SPARK Get Device Status.vi"("MotorControlDevRef in"=w341) -> ("Current"=w340:dbl)  [unwired: 7 in, 3 out]
            n136 = Less?(x=w356, y=-6.0) -> (x < y?=w354:bool)
            n137 = Divide(x=w356, y=-8.857) -> (x/y=w359:dbl)
            n138 = Bundle("Sensor Position"=w356, "Setpoint"=w362) -> (→"Pivot Chart":cluster{"Sensor Position":dbl, "Setpoint":dbl})  [unwired: 1 in]
            n139 = Multiply(x=w359, y="FF multiplier") -> (x*y=w357:dbl)
            n140 = call <vilib>:"SPARK Set Output Advanced.vi"("Arbitrary Feed Forward (0)"=w357, "Control Mode"=Spark_MAX_Control_Type."Position", "Setpoint"=w362, "MotorControlDevRef"=w347) -> ()  [unwired: 6 in, 2 out]
            n141 = call <vilib>:"SPARK Set Output Advanced.vi"("Control Mode"=Spark_MAX_Control_Type."Percent VBus", "Setpoint"=w344, "MotorControlDevRef"=w349) -> ()  [unwired: 7 in, 2 out]
          }
          frame "Coral Intake" {
            # "changed here"
            # "launcher"
            # "funnel"
            # "trapezoid down if we are not at home (0)"
            # "get cascade position"
            # "pivot"
            # "intake until we reach limit switch then launch coral"
            n142 = call-poly <vilib>:"SPARK Get Encoder Status.vi"("MotorControlDevRef in"=w418) -> ("Sensor Position"=w384:dbl, "MotorControlDevRef out"=w417:T11)  [unwired: 7 in, 2 out]
            n143 = call <vilib>:"SPARK Set Output Advanced.vi"("Arbitrary Feed Forward (0)"=w391, "Control Mode"=Spark_MAX_Control_Type."Position", "Setpoint"=0.0, "MotorControlDevRef"=w424) -> ()  [unwired: 6 in, 2 out]
            n144 = call "Deadband Checker.vi"("Limit"=0.9, "Value"=w384) -> ("Outside Deadband?"=w413:bool)  [unwired: 9 in]
            n145 = Index Array(array=w404) -> (element=w402:T23)  [unwired: 1 in]
            n146 = Unbundle(w402) -> ("Trapezoid"=w401:dbl[])  [unwired: 3 out]
            n147 = case shown="True" w413 {
              tunnel: w417 -> [w431 w472]
              tunnel: [w432 w471] -> w407
              tunnel: w384 -> [w432 w470]
              tunnel: "Distance Decrease" -> [_ w469]
              tunnel: [_ w467] -> w403
              tunnel: w401 -> [_ w468]
              tunnel: w400 -> [w430 w466]
              tunnel: w398 -> [_ w465]
              tunnel: w397 -> [_ w464]
              tunnel: w396 -> [_ w462]
              tunnel: [w429 w461] -> w394
              tunnel: [_ w460] -> w392
              frame False {
                n148 = disable-structure shown="Enabled" {
                  disable-tunnel: w431 -> [w435 w457]
                  disable-tunnel: w430 -> [w433 _]
                  disable-tunnel: [_ w456] -> w429
                  frame Disabled {
                    # "changed here"
                    n149 = call <vilib>:"SPARK Set Output Advanced.vi"("Control Mode"=Spark_MAX_Control_Type."Position", "Setpoint"=0.0, "MotorControlDevRef"=w435) -> ("MotorControlDevRef"=w434:T11)  [unwired: 7 in, 1 out]
                    n150 = disable-structure shown="Enabled" {
                      disable-tunnel: w434 -> [w445 _]
                      disable-tunnel: [w438 _] -> _
                      disable-tunnel: w433 -> [w438 _]
                      frame Enabled {
                        w440 = 0.0 ("Setpoint")
                        n151 = for {
                          N: 1 -> [_]
                          tunnel: [w454] -> w447
                          tunnel: w438 -> [w451]
                          shift-right: [w453] -> w446
                          shift-left: w445 -> [w452]
                          w450 = -0.05 ("Setpoint")
                          (unwired) 0.0 ("Position")
                          n152 = call "Arbitrary Feed Forward Generator.vi"("Feed Forward Constants"=w451, "Setpoint"=w450) -> ("Arbitrary Feedforward"=w449:dbl)  [unwired: 9 in]
                          n153 = call <vilib>:"SPARK Set Output Advanced.vi"("Arbitrary Feed Forward (0)"=w449, "Control Mode"=Spark_MAX_Control_Type."Percent VBus", "Setpoint"=w450, "MotorControlDevRef"=w452) -> ("error out"=w454:errorcluster, "MotorControlDevRef"=w453:T11)  [unwired: 6 in]
                          n154 = Wait (ms)(milliseconds to wait=u32 500) -> ()  [unwired: 1 out]
                        }
                        n155 = call "Arbitrary Feed Forward Generator.vi"("Feed Forward Constants"=w438, "Setpoint"=w440) -> ("Arbitrary Feedforward"=w441:dbl)  [unwired: 9 in]
                        n156 = call <vilib>:"SPARK Set Sensor Position.vi"("error in"=w447, "Position"=0.0, "MotorControlDeviceRef"=w446) -> ("MotorControlDeviceRef"=w443:T11)  [unwired: 7 in, 1 out]
                        n157 = call <vilib>:"SPARK Set Output Advanced.vi"("Arbitrary Feed Forward (0)"=w441, "Control Mode"=Spark_MAX_Control_Type."Percent VBus", "Setpoint"=w440, "MotorControlDevRef"=w443) -> ()  [unwired: 6 in, 2 out]
                      }
                      frame Disabled {
                      }
                    }
                  }
                  frame Enabled {
                    n158 = call <vilib>:"SPARK Set Output Advanced.vi"("Control Mode"=Spark_MAX_Control_Type."Percent VBus", "Setpoint"=0.0, "MotorControlDevRef"=w457) -> ("MotorControlDevRef"=w456:T11)  [unwired: 7 in, 1 out]
                  }
                }
              }
              frame True {
                n159 = disable-structure shown="Enabled" {
                  disable-tunnel: w472 -> [w501 w522]
                  disable-tunnel: [w495 w524] -> w471
                  disable-tunnel: w470 -> [_ _]
                  disable-tunnel: w469 -> [_ _]
                  disable-tunnel: [w496 w523] -> w467
                  disable-tunnel: w468 -> [w494 w521]
                  disable-tunnel: w466 -> [w499 w519]
                  disable-tunnel: [w500 w518] -> w463
                  disable-tunnel: w465 -> [w498 _]
                  disable-tunnel: w464 -> [w497 _]
                  disable-tunnel: w462 -> [w493 _]
                  disable-tunnel: [w492 _] -> w460
                  frame Enabled {
                    n160 = case shown="False" w493 {
                      tunnel: w501 -> [w510 w515]
                      tunnel: [w509 w512] -> w500
                      tunnel: w499 -> [w508 w514]
                      tunnel: w498 -> [w507 _]
                      tunnel: w497 -> [w506 _]
                      tunnel: [w504 w513] -> w496
                      tunnel: [w505 w511] -> w495
                      tunnel: w494 -> [_ w516]
                      tunnel: [w503 _] -> w492
                      frame False {
                        n161 = call "Trapezoid on the Fly.vi"("FeedForward Constants"=w508, "Setpoint"=0.6, "Acceleration Max"=w506, "Velocity Max"=w507, "MotorControlDevRef in"=w510) -> ("End Time"=w503:dbl, "Sensor Position"=w505:dbl, "MotorControlDevRef out"=w509:T11, "charted V"=w504:cluster{"Sensor Velocity":dbl, "Numeric":dbl}[])  [unwired: 1 out]
                      }
                      frame True {
                        n162 = Negate(x=w516) -> (-x=w517:dbl[])
                        n163 = call "Apply Trapezoid.vi"("FeedForward Constants"=w514, "Velocity values"=w517, "MotorControlDeviceRef in"=w515) -> ("Sensor Position"=w511:dbl, "MotorControlDevRef out"=w512:T11, "charted V"=w513:cluster{"Sensor Velocity":dbl, "Numeric":dbl}[])  [unwired: 5 in, 1 out]
                      }
                    }
                  }
                  frame Disabled {
                    n164 = Negate(x=w521) -> (-x=w520:dbl[])
                    n165 = call "Apply Trapezoid.vi"("FeedForward Constants"=w519, "Velocity values"=w520, "MotorControlDeviceRef in"=w522) -> ("Sensor Position"=w524:dbl, "MotorControlDevRef out"=w518:T11, "charted V"=w523:cluster{"Sensor Velocity":dbl, "Numeric":dbl}[])  [unwired: 5 in, 1 out]
                  }
                }
                n166 = disable-structure shown="Enabled" {
                  disable-tunnel: w466 -> [w477 _]
                  disable-tunnel: w463 -> [w476 _]
                  disable-tunnel: [w474 _] -> w461
                  frame Enabled {
                    w478 = 0.0 ("Setpoint")
                    n167 = disable-structure shown="Enabled" {
                      disable-tunnel: [w483 w491] -> w475
                      disable-tunnel: w477 -> [w482 _]
                      disable-tunnel: w476 -> [w480 w491]
                      frame Disabled {
                        n168 = for {
                          N: 1 -> [_]
                          tunnel: w482 -> [w487]
                          shift-right: [w489] -> w483
                          shift-left: w480 -> [w488]
                          w486 = -0.05 ("Setpoint")
                          (unwired) 0.0 ("Position")
                          n169 = call "Arbitrary Feed Forward Generator.vi"("Feed Forward Constants"=w487, "Setpoint"=w486) -> ("Arbitrary Feedforward"=w485:dbl)  [unwired: 9 in]
                          n170 = call <vilib>:"SPARK Set Output Advanced.vi"("Arbitrary Feed Forward (0)"=w485, "Control Mode"=Spark_MAX_Control_Type."Percent VBus", "Setpoint"=w486, "MotorControlDevRef"=w488) -> ("MotorControlDevRef"=w489:T11)  [unwired: 6 in, 1 out]
                          n171 = Wait (ms)(milliseconds to wait=u32 500) -> ()  [unwired: 1 out]
                        }
                      }
                      frame Enabled {
                      }
                    }
                    n172 = call "Arbitrary Feed Forward Generator.vi"("Feed Forward Constants"=w477, "Setpoint"=w478) -> ()  [unwired: 9 in, 1 out]
                    n173 = call <vilib>:"SPARK Set Output Advanced.vi"("Arbitrary Feed Forward (0)"=0.0, "Control Mode"=Spark_MAX_Control_Type."Position", "Setpoint"=w478, "MotorControlDevRef"=w475) -> ("MotorControlDevRef"=w474:T11)  [unwired: 6 in, 1 out]
                  }
                  frame Disabled {
                  }
                }
              }
            }
            "Intake Trapezoid Chart" <- w403
            n174 = call "Is Value Changed.vim"("value"=w386) -> ("changed or first call?"=w387:bool)
            n175 = And(x=w386, y=w387) -> (x .and. y?=w385:bool)
            n176 = case shown="True" w385 {
              tunnel: w384 -> [_ w426]
              frame False {
              }
              frame True {
                n177 = Format Into String(initial string="Cascade Intaking Sensor Position: ", w426) -> (resulting string=w428:string)  [unwired: 2 in, 1 out]
                n178 = call <vilib>:"WPI_UtilitiesFRC SendMessageToConsole.vi"("Message"=w428) -> ()  [unwired: 14 in, 1 out]
              }
            }
            n179 = call-poly <vilib>:"SPARK Get Device Status.vi"("MotorControlDevRef in"=w394) -> ("Current"=w393:dbl)  [unwired: 7 in, 3 out]
            n180 = disable-structure shown="Enabled" {
              disable-tunnel: "intake setpoint" -> [w536 w603]
              disable-tunnel: w425 -> [w541 w601]
              disable-tunnel: "detected speed (0)" -> [w540 _]
              disable-tunnel: w421 -> [w539 w600]
              disable-tunnel: [w538 w597] -> w420
              disable-tunnel: w419 -> [w537 w598]
              disable-tunnel: w407 -> [w528 w605]
              disable-tunnel: "launcher speed" -> [w533 w599]
              disable-tunnel: w386 -> [w532 w592]
              disable-tunnel: [w531 w596] -> w410
              disable-tunnel: [w525 w595] -> w406
              disable-tunnel: [w527 w593] -> w405
              disable-tunnel: [w526 w594] -> w395
              disable-tunnel: w390 -> [_ _]
              disable-tunnel: w389 -> [_ w591]
              disable-tunnel: w388 -> [_ w590]
              frame Disabled {
                # "cascade lowered?\ntake coral!"
                # "sensed something?\nintake stop (change?)"
                n181 = call "Deadband Checker.vi"("Limit"=0.9 ("upper limit"), "Value"=w528) -> ("Outside Deadband?"=w529:bool)  [unwired: 9 in]
                n182 = Select(t=0.0, s=w529, f=w536) -> (s? t:f=w534:dbl)
                n183 = case shown="True" w532 {
                  tunnel: w541 -> [w545 w580]
                  tunnel: w540 -> [w549 _]
                  tunnel: w539 -> [w552 w578]
                  tunnel: w533 -> [w551 _]
                  tunnel: [w550 TRUE] -> w538
                  tunnel: w537 -> [w548 _]
                  tunnel: w534 -> [w543 w573]
                  tunnel: [w546 1.0] -> w531
                  tunnel: [w544 "sensor speed launcher"] -> w525
                  tunnel: [w543 w573] -> w527
                  tunnel: [w542 w571] -> w526
                  frame False {
                    # "intake"
                    # "intake is set a power"
                    # "just intake no qualms"
                    n184 = case shown="True" w548 {
                      tunnel: w552 -> [w558 w567]
                      tunnel: w551 -> [w555 _]
                      tunnel: [FALSE TRUE] -> w550
                      tunnel: w549 -> [_ w564]
                      tunnel: [5.0 20.0] -> w546
                      tunnel: [w555 w564] -> w544
                      tunnel: [w553 w562] -> w542
                      frame False {
                        # "set norm speed"
                        n185 = disable-structure shown="Enabled" {
                          disable-tunnel: [Spark_MAX_Control_Type."Percent VBus" ("Control Mode") Spark_MAX_Control_Type."Velocity" ("Control Mode")] -> w556
                          frame Disabled {
                          }
                          frame Enabled {
                          }
                        }
                        n186 = call <vilib>:"SPARK Set Output Advanced.vi"("Control Mode"=w556, "Setpoint"=w555, "MotorControlDevRef"=w558) -> ("MotorControlDevRef"=w554:T11)  [unwired: 7 in, 1 out]
                        n187 = call-poly <vilib>:"SPARK Get Encoder Status.vi"("MotorControlDevRef in"=w554) -> ("Sensor Velocity"=w553:dbl)  [unwired: 7 in, 3 out]
                      }
                      frame True {
                        # "todo: previous 1\nexploring cpu usage"
                        # "if it entered the true case set slow 0"
                        # "set launcher to power"
                        n188 = disable-structure shown="Enabled" {
                          disable-tunnel: [Spark_MAX_Control_Type."Percent VBus" ("Control Mode") Spark_MAX_Control_Type."Percent VBus" ("Control Mode")] -> w568
                          frame Enabled {
                          }
                          frame Disabled {
                          }
                        }
                        n189 = call <vilib>:"SPARK Set Output Advanced.vi"("Control Mode"=w568, "Setpoint"=w564, "MotorControlDevRef"=w567) -> ("MotorControlDevRef"=w563:T11)  [unwired: 7 in, 1 out]
                        n190 = call-poly <vilib>:"SPARK Get Encoder Status.vi"("MotorControlDevRef in"=w563) -> ("Sensor Velocity"=w562:dbl)  [unwired: 7 in, 3 out]
                      }
                    }
                    n191 = call <vilib>:"SPARK Set Output Advanced.vi"("Control Mode"=Spark_MAX_Control_Type."Percent VBus", "Setpoint"=w543, "MotorControlDevRef"=w545) -> ()  [unwired: 7 in, 2 out]
                  }
                  frame True {
                    # "funnel"
                    # "logic for limit switch \nfor launcher"
                    n192 = disable-structure shown="Enabled" {
                      disable-tunnel: w578 -> [w587 w588]
                      disable-tunnel: [w584 w588] -> w577
                      frame Disabled {
                        n193 = call-poly <vilib>:"SPARK Configure Limit Switch.vi"("Enabled? (T)"=TRUE, "Polarity (Normally Open)"=Spark_MAX_Limit_Switch_Polarity."Normally Closed", "MotorControlDeviceRef in"=w587) -> ("MotorControlDeviceRef out"=w584:T11)  [unwired: 7 in, 1 out]
                      }
                      frame Enabled {
                      }
                    }
                    n194 = disable-structure shown="Enabled" {
                      disable-tunnel: [Spark_MAX_Control_Type."Percent VBus" ("Control Mode") Spark_MAX_Control_Type."Velocity" ("Control Mode")] -> w579
                      frame Disabled {
                      }
                      frame Enabled {
                      }
                    }
                    n195 = call <vilib>:"SPARK Set Output Advanced.vi"("Control Mode"=Spark_MAX_Control_Type."Percent VBus", "Setpoint"=w573, "MotorControlDevRef"=w580) -> ()  [unwired: 7 in, 2 out]
                    n196 = call <vilib>:"SPARK Set Output Advanced.vi"("Control Mode"=w579, "Setpoint"="sensor speed launcher", "MotorControlDevRef"=w577) -> ("MotorControlDevRef"=w572:T11)  [unwired: 7 in, 1 out]
                    n197 = call-poly <vilib>:"SPARK Get Encoder Status.vi"("MotorControlDevRef in"=w572) -> ("Sensor Velocity"=w571:dbl)  [unwired: 7 in, 3 out]
                  }
                }
                "detect?" <- w532
              }
              frame Enabled {
                n198 = call "Deadband Checker.vi"("Limit"=0.9 ("upper limit"), "Value"=w605) -> ("Outside Deadband?"=w589:bool)  [unwired: 9 in]
                n199 = Select(t=0.0, s=w589, f=w603) -> (s? t:f=w602:dbl)
                n200 = case shown="True" w592 {
                  tunnel: w601 -> [w617 w637]
                  tunnel: w600 -> [w621 w635]
                  tunnel: w599 -> [w612 _]
                  tunnel: [FALSE TRUE] -> w597
                  tunnel: w602 -> [w609 w625]
                  tunnel: [10.0 2.0] -> w596
                  tunnel: [w613 w629] -> w595
                  tunnel: [w610 w622] -> w593
                  tunnel: [w616 w631] -> w594
                  tunnel: w598 -> [_ _]
                  tunnel: w591 -> [_ _]
                  tunnel: w590 -> [w608 w624]
                  tunnel: w589 -> [_ w627]
                  frame False {
                    # "set norm speed"
                    # "intake"
                    # "intake is set a power"
                    # "just intake no qualms"
                    n201 = Select(t=0.0, s=w608, f=w609) -> (s? t:f=w610:dbl)
                    n202 = Select(t=0.0, s=w608, f=w612) -> (s? t:f=w613:dbl)
                    n203 = call <vilib>:"SPARK Set Output Advanced.vi"("Control Mode"=Spark_MAX_Control_Type."Velocity", "Setpoint"=w613, "MotorControlDevRef"=w621) -> ("MotorControlDevRef"=w614:T11)  [unwired: 7 in, 1 out]
                    n204 = call-poly <vilib>:"SPARK Get Encoder Status.vi"("MotorControlDevRef in"=w614) -> ("Sensor Velocity"=w616:dbl)  [unwired: 7 in, 3 out]
                    n205 = call <vilib>:"SPARK Set Output Advanced.vi"("Control Mode"=Spark_MAX_Control_Type."Percent VBus", "Setpoint"=w610, "MotorControlDevRef"=w617) -> ()  [unwired: 7 in, 2 out]
                  }
                  frame True {
                    # "SPARK Set Output Advanced.vifunnel"
                    # "logic for limit switch \nfor launcher"
                    n206 = Or(x=w627, y=w624) -> (x .or. y?=w623:bool)
                    n207 = Select(t=0.0, s=w623, f=w625) -> (s? t:f=w622:dbl)
                    n208 = call <vilib>:"SPARK Set Output Advanced.vi"("Control Mode"=Spark_MAX_Control_Type."Percent VBus", "Setpoint"=w622, "MotorControlDevRef"=w637) -> ()  [unwired: 7 in, 2 out]
                    n209 = Select(t=0.0, s=w623, f="sensor speed launcher 2") -> (s? t:f=w629:dbl)
                    n210 = call <vilib>:"SPARK Set Output Advanced.vi"("Control Mode"=Spark_MAX_Control_Type."Velocity", "Setpoint"=w629, "MotorControlDevRef"=w635) -> ("MotorControlDevRef"=w632:T11)  [unwired: 7 in, 1 out]
                    n211 = call-poly <vilib>:"SPARK Get Encoder Status.vi"("MotorControlDevRef in"=w632) -> ("Sensor Velocity"=w631:dbl)  [unwired: 7 in, 3 out]
                  }
                }
              }
            }
            "Velocity Chart for Tuning" <- w395
          }
          frame "Scoring Sequence" {
            w659 = T10 0 items=["Slot 0", "Slot 1", "Slot 2", "Slot 3"] ("Closed Loop Slot")
            w669 = T10 0 items=["Slot 0", "Slot 1", "Slot 2", "Slot 3"] ("Closed Loop Slot")
            # "disconnected F here"
            # "dead logic"
            # "v max"
            # "done at comp: if you do not see anything \nin sensor right now = true"
            # "final"
            # "initial"
            # "set 0"
            # "llin reg to convert between trapezoid"
            # "watch susizoids"
            # "setting launcher\nto 0 just in case"
            # "make sure conversion factor is correct"
            # "get current position. check if we are starting from ground or from a non setpoint state. if it is from ground, use known values.\notherwise generate a new one. then do position control to correct"
            n212 = call <vilib>:"SPARK Set Output Advanced.vi"("Arbitrary Feed Forward (0)"=w643, "Control Mode"=Spark_MAX_Control_Type."Position", "Setpoint"=0.0, "MotorControlDevRef"=w675) -> ()  [unwired: 6 in, 2 out]
            n213 = call <vilib>:"SPARK Set Output Advanced.vi"("Control Mode"=Spark_MAX_Control_Type."Percent VBus", "Setpoint"=0.0, "MotorControlDevRef"=w681) -> ()  [unwired: 7 in, 2 out]
            n214 = call-poly <vilib>:"NT Read Value.vi"("name"="/CU-DB/E.E. Setpoint") -> ("value"=w662:dbl)  [unwired: 8 in, 2 out]
            n215 = call <vilib>:"SPARK Set Output Advanced.vi"("Control Mode"=Spark_MAX_Control_Type."Percent VBus", "Setpoint"=0.0, "MotorControlDevRef"=w684) -> ()  [unwired: 7 in, 2 out]
            n216 = Index Array(array=w667, index #1=w668, index #2=w658) -> (element #1=w686:T23, element #2=w657:T23)
            n217 = Unbundle(w686) -> ("Position Setpoint"=w654:dbl, "Trapezoid"=w656:dbl[])  [unwired: 2 out]
            n218 = Unbundle(w657) -> ("Position Setpoint"=w655:dbl)  [unwired: 3 out]
            n219 = Subtract(x=w654, y=w655) -> (x-y=w653:dbl)
            n220 = call "Trapezoid Position Converter.vi"("Distance"=w653, "Initial Parameter"=enum16{"Position", "Trapezoid Distance"}."Position") -> ("Transformed Distance"=w651:dbl)  [unwired: 9 in]
            n221 = call "Generator.vi"("Distance"=w651, "Velocity Max"=w649, "Acceleration Max"=w650) -> ("Velocity values"=w648:dbl[])  [unwired: 7 in, 1 out]
            n222 = Equal?(x=w668, y=Scoring_Levels."L4") -> (x = y?=w671:bool)
            n223 = Select(t=w659, s=w671, f=w669) -> (s? t:f=w660:T10)
            n224 = call-poly <vilib>:"SPARK Get Encoder Status.vi"("MotorControlDevRef in"=w679) -> ("Sensor Position"=w665:dbl, "MotorControlDevRef out"=w666:T11)  [unwired: 7 in, 2 out]
            n225 = Not(x=w642) -> (.not. x?=w641:bool)
            n226 = case shown="True" TRUE {
              tunnel: w678 -> [_ w699]
              tunnel: w660 -> [_ _]
              tunnel: w666 -> [w690 w704]
              tunnel: w665 -> [w691 w697]
              tunnel: [w691 w702] -> w664
              tunnel: w649 -> [_ w703]
              tunnel: w650 -> [_ w701]
              tunnel: w654 -> [_ w700]
              tunnel: w656 -> [_ w696]
              tunnel: w648 -> [_ w695]
              tunnel: w647 -> [_ w694]
              tunnel: [w687 w693] -> w646
              tunnel: [_ w692] -> w644
              frame False {
                n227 = call <vilib>:"SPARK Set Output Advanced.vi"("Control Mode"=Spark_MAX_Control_Type."Percent VBus", "Setpoint"=0.0, "MotorControlDevRef"=w690) -> ("MotorControlDevRef"=w687:T11)  [unwired: 7 in, 1 out]
              }
              frame True {
                # "positional correction"
                # "-12.381"
                n228 = disable-structure shown="Enabled" {
                  disable-tunnel: w704 -> [w718 _]
                  disable-tunnel: w703 -> [w717 _]
                  disable-tunnel: [w716 _] -> w702
                  disable-tunnel: w701 -> [w715 _]
                  disable-tunnel: w700 -> [w714 _]
                  disable-tunnel: w699 -> [w708 _]
                  disable-tunnel: [w713 _] -> w698
                  disable-tunnel: w697 -> [w711 _]
                  disable-tunnel: w696 -> [w710 _]
                  disable-tunnel: w695 -> [w709 _]
                  disable-tunnel: w694 -> [w707 _]
                  disable-tunnel: [w706 _] -> w693
                  disable-tunnel: [w705 _] -> w692
                  frame Enabled {
                    n229 = case shown="False" w707 {
                      tunnel: w718 -> [w728 w742]
                      tunnel: w717 -> [w727 _]
                      tunnel: [w726 w732] -> w716
                      tunnel: w715 -> [w725 _]
                      tunnel: w714 -> [w724 w730]
                      tunnel: [w722 w743] -> w713
                      tunnel: [w721 w744] -> w712
                      tunnel: w711 -> [_ w741]
                      tunnel: w710 -> [_ w740]
                      tunnel: w709 -> [_ w738]
                      tunnel: w708 -> [w723 w731]
                      tunnel: [w720 w729] -> w706
                      tunnel: [w719 _] -> w705
                      frame False {
                        n230 = call "Trapezoid on the Fly.vi"("FeedForward Constants"=w723, "Setpoint"=w724, "Acceleration Max"=w725, "Velocity Max"=w727, "MotorControlDevRef in"=w728) -> ("End Time"=w719:dbl, "Post-Trapezoid Sensor Position"=w722:dbl, "Sensor Position"=w726:dbl, "MotorControlDevRef out"=w720:T11, "charted V"=w721:cluster{"Sensor Velocity":dbl, "Numeric":dbl}[])
                      }
                      frame True {
                        w735 = T10 0 items=["Slot 0", "Slot 1", "Slot 2", "Slot 3"] ("Closed Loop Slot")
                        n231 = call "Deadband Checker.vi"("Limit"=1.5, "Value"=w741) -> ("Outside Deadband?"=w745:bool)  [unwired: 9 in]
                        n232 = Not(x=w745) -> (.not. x?=w747:bool)
                        n233 = Select(t=w740, s=w747, f=w738) -> (s? t:f=w739:dbl[])
                        n234 = call "Apply Trapezoid.vi"("FeedForward Constants"=w731, "Velocity values"=w739, "MotorControlDeviceRef in"=w742) -> ("Sensor Position"=w743:dbl, "MotorControlDevRef out"=w737:T11, "charted V"=w744:cluster{"Sensor Velocity":dbl, "Numeric":dbl}[])  [unwired: 5 in, 1 out]
                        n235 = call "Arbitrary Feed Forward Generator.vi"("Feed Forward Constants"=w731, "Setpoint"=w730) -> ("Arbitrary Feedforward"=w736:dbl)  [unwired: 9 in]
                        n236 = call <vilib>:"SPARK Set Output Advanced.vi"("Arbitrary Feed Forward (0)"=w736, "Closed Loop Slot"=w735, "Control Mode"=Spark_MAX_Control_Type."Position", "Setpoint"=w730, "MotorControlDevRef"=w737) -> ("MotorControlDevRef"=w733:T11)  [unwired: 5 in, 1 out]
                        n237 = call-poly <vilib>:"SPARK Get Encoder Status.vi"("MotorControlDevRef in"=w733) -> ("Sensor Position"=w732:dbl, "MotorControlDevRef out"=w729:T11)  [unwired: 7 in, 2 out]
                      }
                    }
                    "Scoring Sequence Trapezoid" <- w712
                  }
                  frame Disabled {
                    w755 = T10 0 items=["Slot 0", "Slot 1", "Slot 2", "Slot 3"] ("Closed Loop Slot")
                    n238 = call "Arbitrary Feed Forward Generator.vi"() -> ("Arbitrary Feedforward"=w749:dbl, "Setpoint"=w748:dbl)  [unwired: 10 in]
                    n239 = call <vilib>:"SPARK Set Output Advanced.vi"("Arbitrary Feed Forward (0)"=w749, "Closed Loop Slot"=w755, "Control Mode"=Spark_MAX_Control_Type."Position", "Setpoint"=w748) -> (3:"MotorControlDevRef"=w753:T11, 11:"MotorControlDevRef"=w756:T11)  [unwired: 5 in, 1 out]
                    n240 = call-poly <vilib>:"SPARK Get Encoder Status.vi"("MotorControlDevRef in"=w753) -> ("Sensor Position"=w751:dbl)  [unwired: 7 in, 3 out]
                    n241 = Bundle("Sensor Position"=w751) -> (w752:cluster{"Sensor Position":dbl, void}, w750)  [unwired: 1 in]
                  }
                }
                "Post-Trapezoid Sensor Position" <- w698
              }
            }
            "Post Position Correction" <- w664
            n242 = call-poly <vilib>:"SPARK Get Device Status.vi"("MotorControlDevRef in"=w646) -> ("Current"=w645:dbl)  [unwired: 7 in, 3 out]
          }
          frame "Score" {
            w775 = T10 0 items=["Slot 0", "Slot 1", "Slot 2", "Slot 3"] ("Closed Loop Slot")
            # "launcher"
            # "coral LAUNCH"
            n243 = Index Array(array=w772, index=w771) -> (element=w770:T23)
            n244 = call "Arbitrary Feed Forward Generator.vi"("Feed Forward Constants"=w776) -> ("Arbitrary Feedforward"=w777:dbl)  [unwired: 10 in]
            n245 = Unbundle(w770) -> ("Position Setpoint"=w768:dbl, "Score Power"=w762:dbl)  [unwired: 2 out]
            n246 = call <vilib>:"SPARK Set Output Advanced.vi"("Arbitrary Feed Forward (0)"=w777, "Closed Loop Slot"=w775, "Control Mode"=Spark_MAX_Control_Type."Position", "Setpoint"=w768, "MotorControlDevRef"=w769) -> ("MotorControlDevRef"=w767:T11)  [unwired: 5 in, 1 out]
            n247 = call-poly <vilib>:"SPARK Get Encoder Status.vi"("MotorControlDevRef in"=w767) -> ("Sensor Position"=w763:dbl, "MotorControlDevRef out"=w758:T11)  [unwired: 7 in, 2 out]
            n248 = call <vilib>:"SPARK Set Output Advanced.vi"("Control Mode"=Spark_MAX_Control_Type."Percent VBus", "Setpoint"=w762, "MotorControlDevRef"=w766) -> ()  [unwired: 7 in, 2 out]
            n249 = call-poly <vilib>:"SPARK Get Device Status.vi"("MotorControlDevRef in"=w758) -> ("Current"=w757:dbl)  [unwired: 7 in, 3 out]
            n250 = call-poly <vilib>:"NT Read Value.vi"("name"="/CU-DB/Intake Setpoint") -> ("value"=w760:dbl)  [unwired: 8 in, 2 out]
          }
          frame "Manual Override" {
            w789 = 0.2 ("t")
            # "set power to control cascade"
            n251 = Negate(x=w789) -> (-x=w788:dbl)
            n252 = Select(t=w788, s=w799, f=w789) -> (s? t:f=w795:dbl)
            n253 = call "Arbitrary Feed Forward Generator.vi"("Feed Forward Constants"=w796, "Setpoint"=w795) -> ("Arbitrary Feedforward"=w797:dbl)  [unwired: 9 in]
            n254 = call <vilib>:"SPARK Set Output Advanced.vi"("Arbitrary Feed Forward (0)"=w797, "Control Mode"=Spark_MAX_Control_Type."Percent VBus", "Setpoint"=w795, "MotorControlDevRef"=w800) -> ("MotorControlDevRef"=w791:T11)  [unwired: 6 in, 1 out]
            n255 = call-poly <vilib>:"SPARK Get Encoder Status.vi"("MotorControlDevRef in"=w791) -> ("Sensor Position"=w787:dbl, "MotorControlDevRef out"=w781:T11)  [unwired: 7 in, 2 out]
            n256 = call-poly <vilib>:"SPARK Get Device Status.vi"("MotorControlDevRef in"=w781) -> ("Current"=w780:dbl)  [unwired: 7 in, 3 out]
            n257 = call-poly <vilib>:"NT Read Value.vi"("name"="/CU-DB/Intake Setpoint") -> ("value"=w783:dbl)  [unwired: 8 in, 2 out]
            n258 = call-poly <vilib>:"NT Read Value.vi"("name"="/CU-DB/E.E. Setpoint") -> ("value"=w785:dbl)  [unwired: 8 in, 2 out]
          }
          frame "Hold Position" {
            w803 = T10 0 items=["Slot 0", "Slot 1", "Slot 2", "Slot 3"] ("Closed Loop Slot")
            w827 = T10 0 items=["Slot 0", "Slot 1", "Slot 2", "Slot 3"] ("Closed Loop Slot")
            # "this should be false"
            # "cascade"
            # "suspect"
            # "hold whatever positon you are at after manual override or scoring sequence"
            n259 = Index Array(array=w821, index=w820) -> (element=w819:T23)
            n260 = Unbundle(w819) -> ("Position Setpoint"=w818:dbl)  [unwired: 3 out]
            n261 = Not(x=w810) -> (.not. x?=w809:bool)
            n262 = And(x=w809, y=w808) -> ()  [unwired: 1 out]
            n263 = call-poly <vilib>:"SPARK Get Encoder Status.vi"("MotorControlDevRef in"=w830) -> ("Sensor Position"=w826:dbl, "MotorControlDevRef out"=w825:T11)  [unwired: 7 in, 2 out]
            n264 = call <vilib>:"SPARK Set Output Advanced.vi"("Arbitrary Feed Forward (0)"=w804, "Closed Loop Slot"=w827, "Control Mode"=Spark_MAX_Control_Type."Position", "Setpoint"=w826, "MotorControlDevRef"=w825) -> ()  [unwired: 5 in, 2 out]
            n265 = call "Arbitrary Feed Forward Generator.vi"("Feed Forward Constants"=w828, "Setpoint"=w826) -> ("Arbitrary Feedforward"=w801:dbl)  [unwired: 9 in]
            n266 = Equal?(x=Scoring_Levels."L4" ("y"), y=w820) -> ()  [unwired: 1 out]
            n267 = call-poly <vilib>:"SPARK Get Encoder Status.vi"("MotorControlDevRef in"=w831) -> ("Sensor Position"=w815:dbl, "MotorControlDevRef out"=w832:T11)  [unwired: 7 in, 2 out]
            n268 = call <vilib>:"SPARK Set Output Advanced.vi"("Arbitrary Feed Forward (0)"=w801, "Closed Loop Slot"=w803, "Control Mode"=Spark_MAX_Control_Type."Position", "Setpoint"=w818, "MotorControlDevRef"=w832) -> ("MotorControlDevRef"=w806:T11)  [unwired: 5 in, 1 out]
            n269 = call-poly <vilib>:"SPARK Get Device Status.vi"("MotorControlDevRef in"=w806) -> ("Current"=w805:dbl)  [unwired: 7 in, 3 out]
            n270 = call-poly <vilib>:"NT Read Value.vi"("name"="/CU-DB/E.E. Setpoint") -> ("value"=w813:dbl)  [unwired: 8 in, 2 out]
            n271 = call-poly <vilib>:"NT Read Value.vi"("name"="/CU-DB/Intake Setpoint") -> ("value"=w811:dbl)  [unwired: 8 in, 2 out]
          }
        }
        "Current" <- w181
        "End Time" <- w180
        n272 = feedback-in #5(w186) -> ()
        n273 = feedback-in #6(w206) -> ()
        n274 = Bundle("Sensor Position"=w201) -> (→"Position Chart (All Time)":cluster{"Sensor Position":dbl})  [unwired: 1 in]
        n275 = global write "Robot Global Data.vi" "Can Climb?"(w207) -> ()
        n276 = call-poly <vilib>:"NT Write Value.vi"("value"=w192, "name"="/CU-DB/Cascade Sensor") -> ()  [unwired: 9 in, 1 out]
        n277 = call-poly <vilib>:"NT Write Value.vi"("value"=w191, "name"="/CU-DB/E.E. Setpoint") -> ()  [unwired: 9 in, 1 out]
        n278 = call-poly <vilib>:"NT Write Value.vi"("value"=w188, "name"="/CU-DB/Intake Setpoint") -> ()  [unwired: 9 in, 1 out]
      }
      frame "Calibrate" {
        # "set cascade/pivot to 0"
        n279 = call <vilib>:"SPARK Set Output Advanced.vi"("Control Mode"=Spark_MAX_Control_Type."Percent VBus", "Setpoint"=0.0, "MotorControlDevRef"=w838) -> ()  [unwired: 7 in, 2 out]
        n280 = call <vilib>:"SPARK Set Output Advanced.vi"("Control Mode"=Spark_MAX_Control_Type."Percent VBus", "Setpoint"=0.0, "MotorControlDevRef"=w835) -> ()  [unwired: 7 in, 2 out]
        n281 = call <vilib>:"SPARK Set Sensor Position.vi"("Position"=0.0, "MotorControlDeviceRef"=w844) -> ()  [unwired: 8 in, 2 out]
        n282 = call <vilib>:"SPARK Set Sensor Position.vi"("Position"=0.0, "MotorControlDeviceRef"=w839) -> ()  [unwired: 8 in, 2 out]
      }
      frame "Reserve" {
        w860 = -1.0  # Infinite
        # "because it foundationally does the same thing as reserve"
        # "set comment or print to say you should NOT want to be in here"
        # "If loop needs to poll sensors or other\nvalues, use a timeout value. -1 waits for\nnext command to be sent."
        n283 = call-poly <vilib>:"SPARK Get Encoder Status.vi"("MotorControlDevRef in"=w855) -> ("Sensor Position"=w856:dbl, "MotorControlDevRef out"=w857:T11)  [unwired: 7 in, 2 out]
        n284 = call-poly <vilib>:"SPARK Get Encoder Status.vi"("MotorControlDevRef in"=w845) -> ("Sensor Position"=w846:dbl, "MotorControlDevRef out"=w847:T11)  [unwired: 7 in, 2 out]
        n285 = call <vilib>:"SPARK Set Output Advanced.vi"("Control Mode"=Spark_MAX_Control_Type."Percent VBus", "Setpoint"=0.0, "MotorControlDevRef"=w854) -> ()  [unwired: 7 in, 2 out]
        n286 = call <vilib>:"SPARK Set Output Advanced.vi"("Control Mode"=Spark_MAX_Control_Type."Position", "Setpoint"=w856, "MotorControlDevRef"=w857) -> ()  [unwired: 7 in, 2 out]
        n287 = call <vilib>:"SPARK Set Output Advanced.vi"("Control Mode"=Spark_MAX_Control_Type."Position", "Setpoint"=w846, "MotorControlDevRef"=w847) -> ()  [unwired: 7 in, 2 out]
        n288 = call <vilib>:"SPARK Set Output Advanced.vi"("Control Mode"=Spark_MAX_Control_Type."Percent VBus", "Setpoint"=0.0, "MotorControlDevRef"=w849) -> ()  [unwired: 7 in, 2 out]
      }
    }
    n289 = call "Coral Check for New Command.vi"("Current Command"=w140, "Wait time (ms)"=w145, "Finished?"=w146) -> ("Completion"=w141:T7, "Subsystem Name"=w142:string, "Current Command"=w143:T3, "Initial Trace String"=w144:string, "NextCommand"=w147:T18)  [unwired: 4 in]
    n290 = case shown="\"Successful\", \"Aborted\"" w141 {
      selector: w141 -> [_ w868]
      tunnel: w144 -> [_ w864]
      tunnel: w143 -> [_ w865]
      tunnel: w142 -> [_ w861]
      frame "Incomplete", Default {
        # "Continuing current command"
      }
      frame "Successful", "Aborted" {
        # "Report and setup for next command"
        n291 = Unbundle By Name(w865) -> ("Coral States"=w867:T5, "Setpoint State"=w862:T6)
        n292 = Format Into String(format string="CS %s, SS %s", initial string=w864, w867, w862) -> (resulting string=w863:string)  [unwired: 1 in, 1 out]
        "Current\nCmd" <- w863
        n293 = call <vilib>:"Trace Results.vi"("Status of previous command"=w868, "Description"=w863, "Subsystem"=w861) -> ()  [unwired: 9 in]
      }
    }
    n294 = disable-structure shown="Enabled" {
      frame Disabled {
        # "Publish"
        n295 = call-poly <vilib>:"NT Write Value.vi"() -> ()  [unwired: 11 in, 1 out]
      }
      frame Enabled {
      }
    }
  }
